vi "ProdaNG.Configurator.vi"() -> ()   [LabVIEW 2016]
uses:
  ProdaNG.Tree.TestViewMode.ctl
  ProdaNG.File.Sequence.ctl
  ProdaNG.Tree.Fglb.Value.ctl
  ProdaNG.File.Step.ctl
  ProdaNG.Configurator.DB.ctl
  ProdaNG.Configurator.Config.ctl
  ProdaNG.Configurator.ResultsTimeSpan.ctl
  Controls/ProdaNG.Product.ctl
  ProdaNG.Configurator.State.ctl
  <vilib>/Utility/error.llb/DialogTypeEnum.ctl
  <vilib>/Utility/miscctls.llb/LVNodeAndColumnTypeDef.ctl
  ProdaNG.Configurator.Glb.vi
panel:
  out "Products":T1[](array[typedef])
  out "DBtime":timestamp
  out "SelectedFile":path
  out "Progress":bool caption="Please wait..."
  out "Hider":bool
  out "PrevTabState":i32
  in  "ButtonResults":bool
  out "SlotInUse":i32
  in  "ButtonTest":bool
  in  "ButtonParts":bool
  out "DB":T2
  out "ProfInfo":string[](array[string])
  in  "TestTreeView":T3
  out "FPref":refnum<vi>
  out "FileContent":T4
  in  "MainTab":enum32{"Parts", "Test", "Results"}(tab)
  in  "ButtonConnect":bool caption="Check"
  out "HiderParts":bool
  in  "ButtonGoToResults":bool
  in  "ButtonGoToTest":bool caption="Accept"
  in  "VariantFilter":string caption="Wabco Part Filter"
  in  "ButtonRefreshTreeProc":bool caption="Refresh"
  in  "ProcTree":string(tree) caption="Found 31 wabco parts"
  out "Identification":T7
  out "Process Found":bool
  in  "color legend 4":u32(colorbox)=16448250 caption="- wabco part"
  in  "color legend 5":u32(colorbox)=12058551 caption="- process"
  in  "color legend 6":u32(colorbox)=16777134 caption="- process step"
  in  "ButtonReloadDB":bool caption="Refresh"
  in  "Configuration":T8={"ShowUnreleased"=TRUE, "Param1"="StepIndex", "ParamStartIdx"=0, "Slots"=1} {"Slots" min=1 max=2; "ParamStartIdx" min=0 max=1}
  in  "TestTree.OpenCloseAll":bool caption="collapse all"
  in  "ButtonSaveToFile":bool
  out "FileInUse":string caption="No file selected"
  in  "ButtonCloseFile":bool
  in  "ButtonExportFile":bool
  in  "ButtonOpenFile":bool
  in  "color legend 1":u32(colorbox)=16448250 caption="- item synchronized"
  in  "color legend 3":u32(colorbox)=16744576 caption="- item value changed"
  in  "color legend 2":u32(colorbox)=16777147 caption="- new item in file (not found in DB)"
  in  "ButtonUnreleaseAll":bool
  in  "ButtonReleaseAll":bool
  in  "ButtonUnrelease":bool
  in  "ButtonRelease":bool
  in  "ButtonDeleteAll":bool
  in  "ButtonAdd":bool
  in  "ButtonEdit":bool
  in  "ButtonDelete":bool
  in  "TestTree":string[](tree)
  in  "ButtonRefreshTestTree":bool
  in  "ResultsAmount":i32=1 caption="Span" min=1 max=100
  in  "ResultsSpan":T9
  in  "Results.TimeTo":timestamp caption="Time To" format="%<%x %X>T"
  in  "Results.TimeFrom":timestamp caption="Time From" format="%<%x %X>T"
  in  "ProductList":i32[](listbox) caption="Products #1"
  in  "color legend 9":u32(colorbox)=16448250 caption="- value ok"
  in  "color legend 8":u32(colorbox)=16744576 caption="- value nok"
  in  "color legend 7":u32(colorbox)=13816530 caption="- value missing"
  in  "ResultsTree":string[](tree)
  in  "ButtonRefreshResultTree":bool
  in  "ProductListSelectAll":enum8{"False", "True", "Mixed"}(c332) caption="All"
  in  "Starthere":bool
  out "Status":string
  out "DBStatus":string
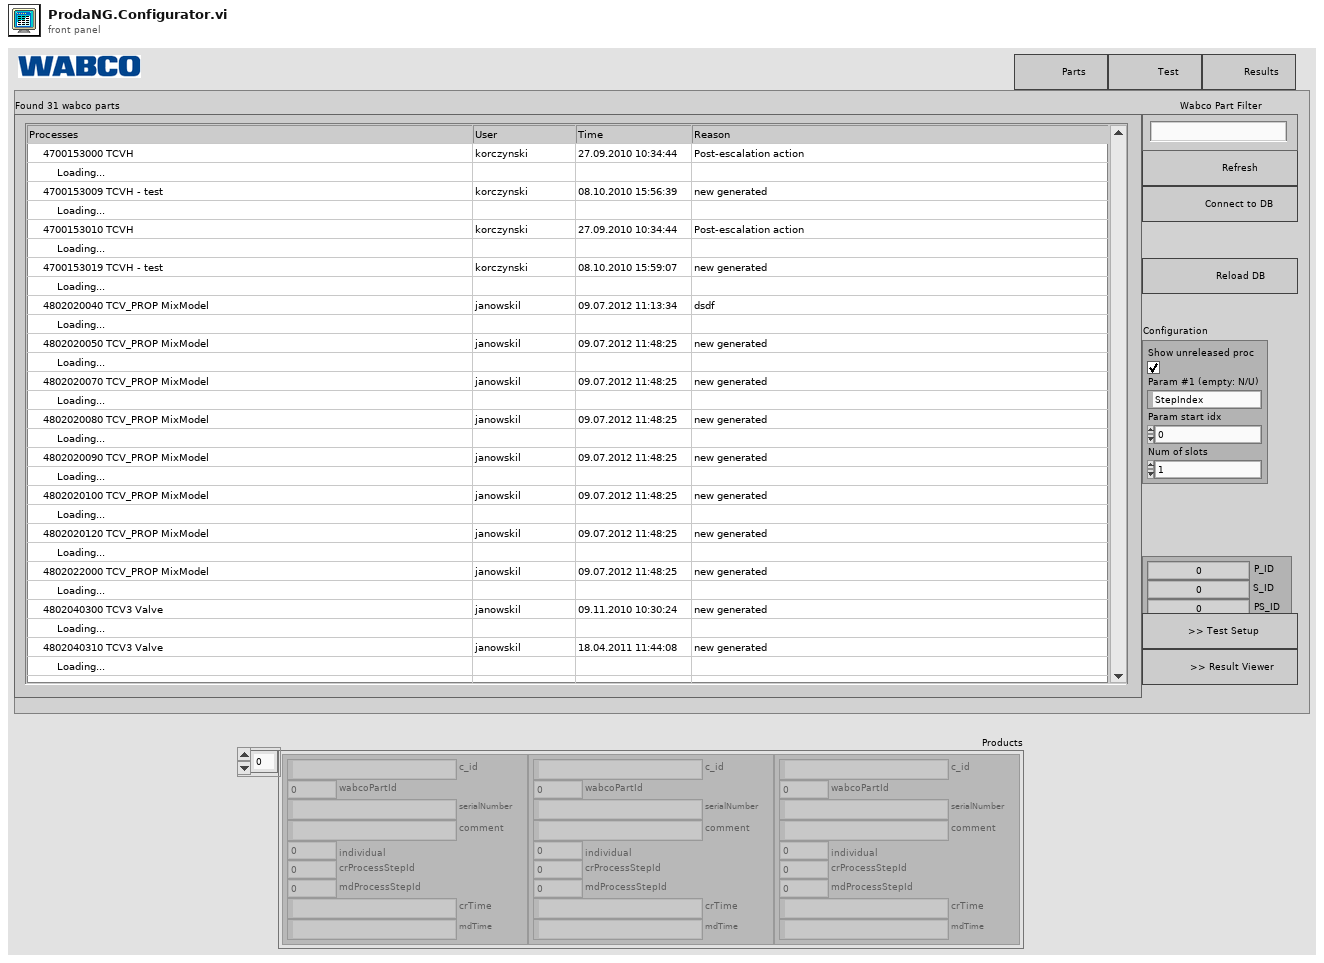
[diagram p1: front panel]
types:
  T1 = typedef "ProdaNG.Product.ctl" = cluster{"c_id":string, "wabcoPartId":i32, "serialNumber":string, "comment":string, "individual":i32, "crProcessStepId":i32, "mdProcessStepId":i32, "crTime":string, "mdTime":string}
  T2 = typedef "ProdaNG.Configurator.DB.ctl" = enum16{"other", "WPL", "WPK"}
  T3 = typedef "ProdaNG.Tree.TestViewMode.ctl" = enum16{"All", "Released", "Unreleased"}
  T4 = typedef "ProdaNG.File.Sequence.ctl" = cluster{"PP":T5[], "TS":T6[]}
  T5 = typedef "ProdaNG.Tree.Fglb.Value.ctl" = cluster{"desc":string, "order":i32, "value1":dbl, "value2":dbl, "unit":i32}
  T6 = typedef "ProdaNG.File.Step.ctl" = cluster{"TS":T5, "TP":T5[], "TV":T5[]}
  T7 = cluster{"P_ID":i32, "S_ID":i32, "PS_ID":i32, "WP_ID":i32}
  T8 = typedef "ProdaNG.Configurator.Config.ctl" = cluster{"ShowUnreleased":bool, "Param1":string, "ParamStartIdx":i32, "Slots":i32}
  T9 = typedef "ProdaNG.Configurator.ResultsTimeSpan.ctl" = enum16{"Custom", "Shift(s)", "Hour(s)", "Day(s)", "Week(s)", "Month(s)"}
  T10 = typedef "ProdaNG.Configurator.State.ctl" = enum16{"Disconnected", "Connected", "ProcessFound"}
  T11 = enum32{"invalid app kind", "Development System", "Run Time System", "Student Edition", "Embedded LabVIEW", "Evaluation", "Custom"}
  T12 = enum8{"Enabled", "Disabled", "Disabled and Grayed Out"}
  T13 = cluster{"processId":i32, "systemId":i32, "processStepId":i32, "wabcoPartId":i32}
  T14 = typedef "DialogTypeEnum.ctl" = enum16{"no dialog", "OK message", "continue or stop message", "auto error handling dialog", "OK message + warnings", "continue/stop + warnings"}
  T15 = typedef "LVNodeAndColumnTypeDef.ctl" = cluster{"Node":string, "Column":i32}
  T16 = enum16{"Custom", "Shift(s)", "Hour(s)", "Day(s)", "Week(s)", "Month(s)"}
  T17 = typedef "LVPositionTypeDef.ctl" = cluster{"Left":i32, "Top":i32}
  T18 = typedef "ProdaNG.ProdutionLine.ctl" = cluster{"i_id":i32, "description":string}
  T19 = typedef "ProdaNG.System.ctl" = cluster{"i_id":i32, "description":string}
  T20 = typedef "ProdaNG.Process.ctl" = cluster{"i_id":i32, "productionLineId":i32, "releaseId":i32, "contentId":string, "previewId":string, "mdReason":string, "mdUser":string, "mdTime":string, "description":string}
  T21 = typedef "ProdaNG.WabcoPart.ctl" = cluster{"i_id":i32, "workCenterId":i32, "contentId":string, "previewId":string, "mdReason":string, "mdUser":string, "mdTime":string, "productName":string, "wabcoNumber":string}
  T22 = typedef "ProdaNG.ProcessStep.ctl" = cluster{"i_id":i32, "processId":i32, "systemId":i32, "releaseId":i32, "processSequence":i32, "limitYellow":dbl, "limitRed":dbl, "mdReason":string, "mdUser":string, "mdTime":string, "filename":string, "transfer":string, "description":string}
  T23 = typedef "ProdaNG.Tree.Fglb.Data.ctl" = cluster{"tag":string, "row":i32, "element":T24, "idx1":i32, "idx2":i32, "file":bool}
  T24 = typedef "ProdaNG.Tree.Fglb.Element.ctl" = enum16{"-", "PP", "TS", "TP", "TV"}
  T25 = typedef "ProdaNG.UnitSimple.ctl" = cluster{"name":string, "i_id":i32}
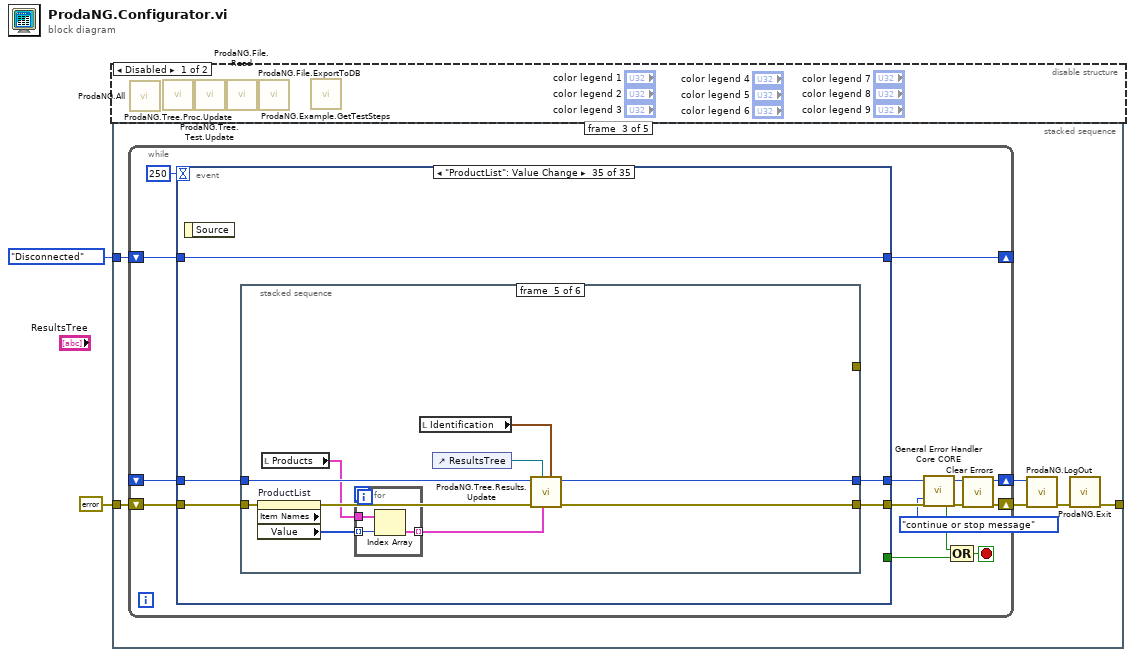
[diagram p0: block diagram]
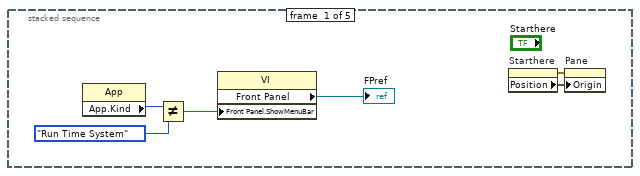
[diagram p2: hidden frame]
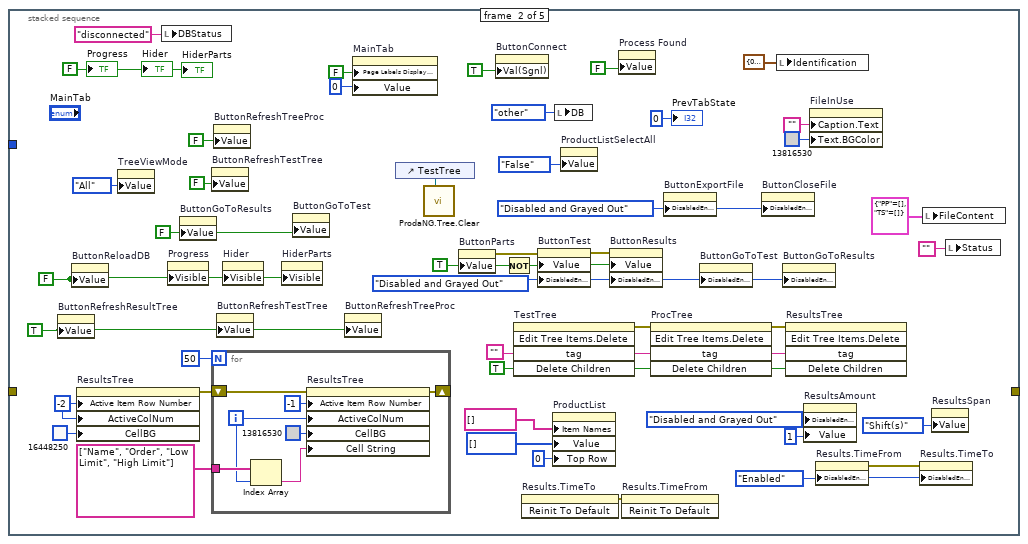
[diagram p3: hidden frame]
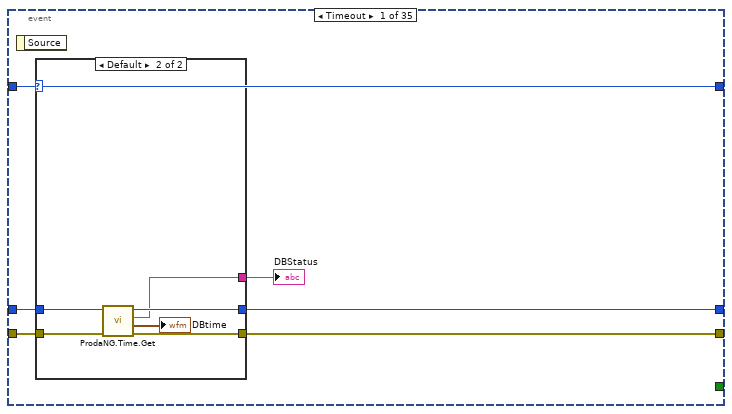
[diagram p4: hidden frame]
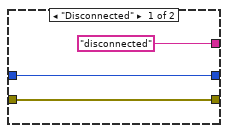
[diagram p5: hidden frame]
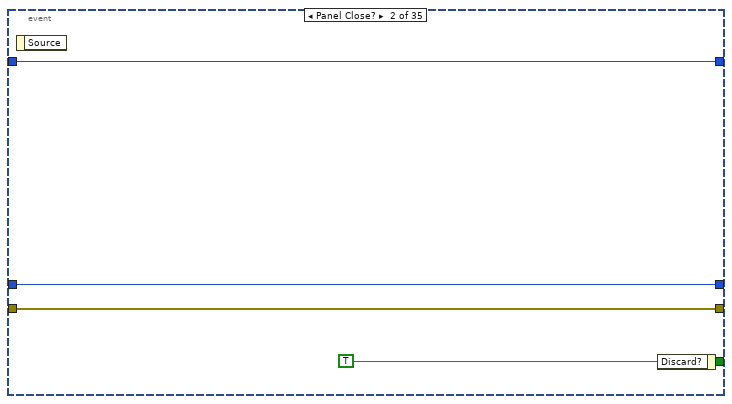
[diagram p6: hidden frame]
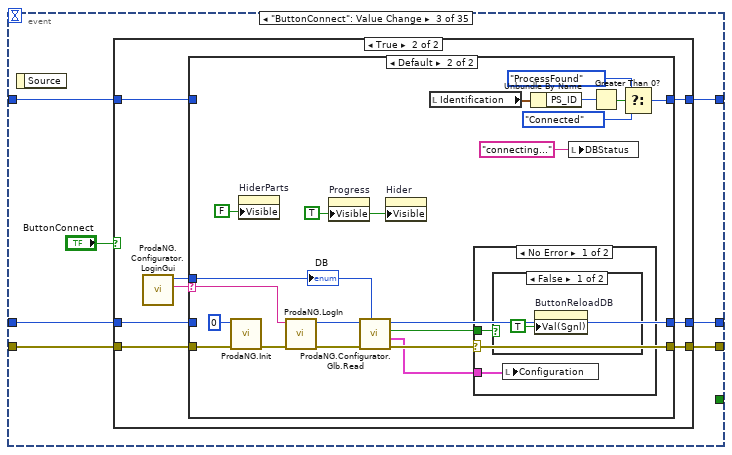
[diagram p7: hidden frame]
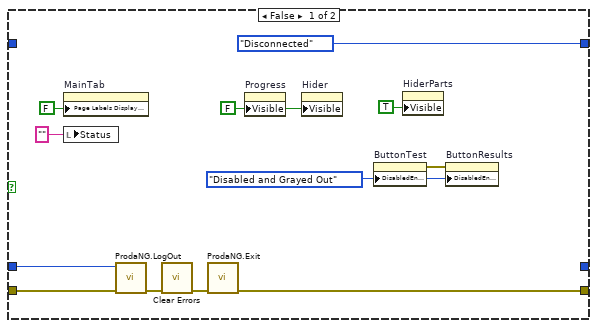
[diagram p8: hidden frame]
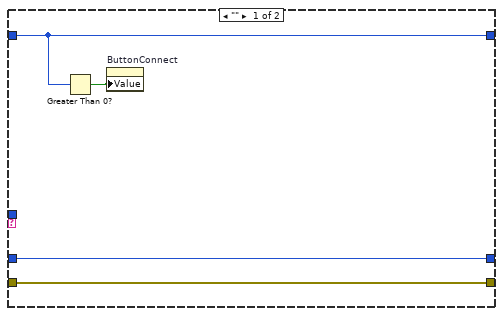
[diagram p9: hidden frame]
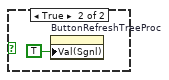
[diagram p10: hidden frame]
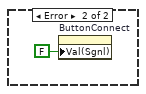
[diagram p11: hidden frame]
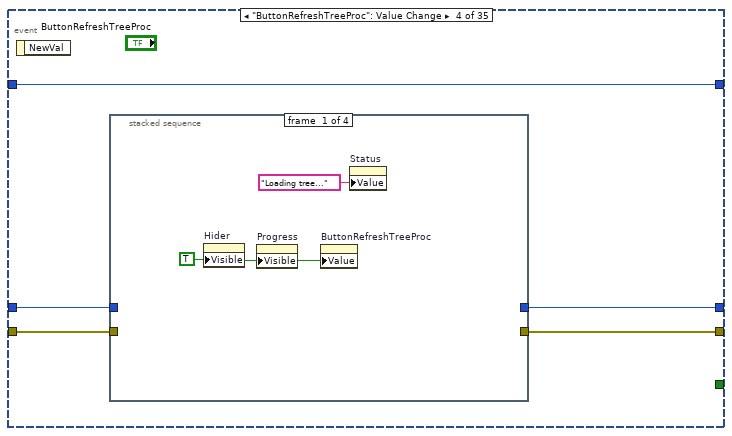
[diagram p12: hidden frame]
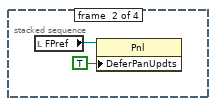
[diagram p13: hidden frame]
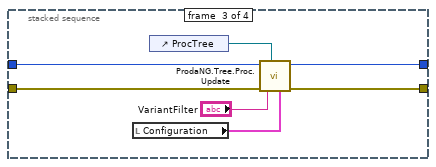
[diagram p14: hidden frame]
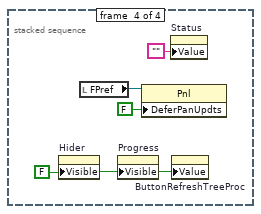
[diagram p15: hidden frame]
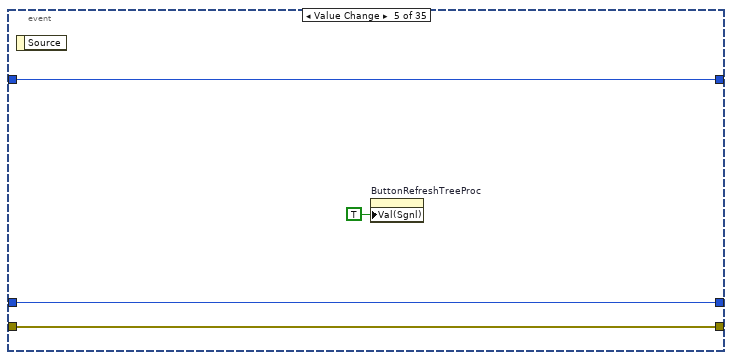
[diagram p16: hidden frame]
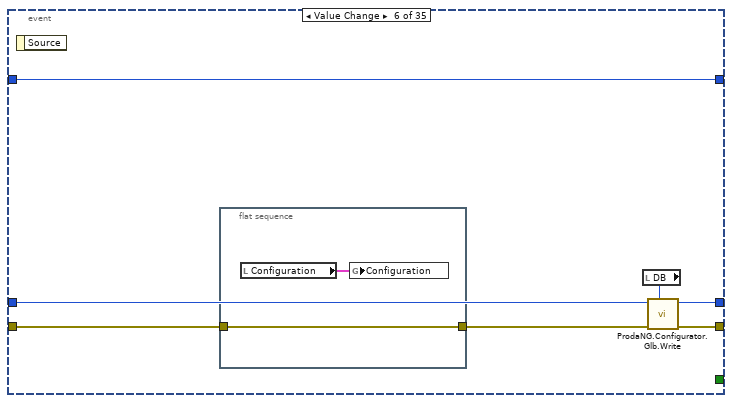
[diagram p17: hidden frame]
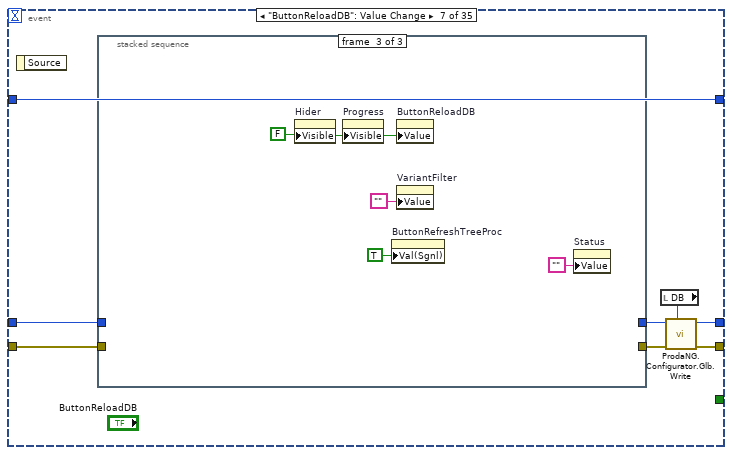
[diagram p18: hidden frame]
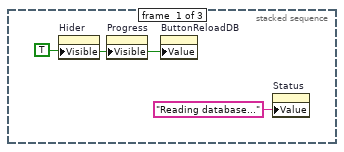
[diagram p19: hidden frame]
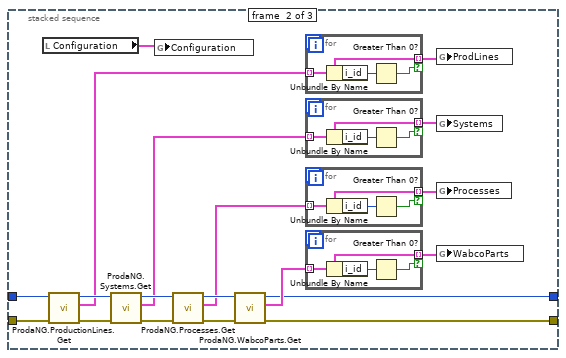
[diagram p20: hidden frame]
diagram:
  n1 = disable-structure shown="Disabled" {
    frame Disabled {
      n2 = call "ProdaNG.All.vi"() -> ()  [unwired: 1 in]
      n3 = call "ProdaNG.Tree.Proc.Update.vi"() -> ()  [unwired: 10 in, 2 out]
      n4 = call "ProdaNG.Tree.Test.Update.vi"() -> ()  [unwired: 8 in, 4 out]
      n5 = call "ProdaNG.File.Read.vi"() -> ()  [unwired: 9 in, 3 out]
      n6 = call "ProdaNG.File.ExportToDB.vi"() -> ()  [unwired: 10 in, 2 out]
      n7 = call "ProdaNG.Example.GetTestSteps.vi"() -> ()  [unwired: 12 in]
    }
    frame Enabled {
    }
  }
  n8 = stacked-sequence {
    tunnel: ProdaNG.Configurator.State."Disconnected" ("State") -> [_ _ w64 _ _]
    tunnel: [_ _ w62 _ _] -> _
    tunnel: errorcluster {"status"=FALSE, "code"=0, "source"=""} ("error out") -> [_ _ w61 _ _]
    frame #0 {
      n9 = property class="App"() -> ("App.Kind"=w8:T11)  [unwired: 2 in, 2 out]
      n10 = Not Equal?(x=w8, y=T11."Run Time System") -> (x != y?=w5:bool)
      n11 = property class="VI"("Front Panel.ShowMenuBar"=w5) -> ("Front Panel"=→"FPref":refnum<vi>)  [unwired: 2 in, 2 out]
      n12 = property on="Starthere" class="Bool (strict)"() -> (error out=w4:errorcluster, "Position"=w3:T17)  [unwired: 2 in, 1 out]
      n13 = property on="Pane" class="Pane"(error in=w4, "Origin"=w3) -> ()  [unwired: 1 in, 2 out]
    }
    frame #1 {
      w11 = T12."Enabled" ("Disabled")
      w15 = TRUE ("Value (Signaling)")
      w21 = -2 ("Active Item:Row Number")
      w26 = TRUE ("Delete Children?")
      w27 = ""
      w31 = FALSE ("Progress")
      w32 = FALSE ("ButtonGoToResults")
      w34 = T12."Disabled and Grayed Out" ("Disabled")
      w39 = TRUE ("ButtonPartList")
      w30 = FALSE ("Visible")
      w47 = T12."Disabled and Grayed Out" ("Disabled")
      n14 = property on="ButtonRefreshResultTree" class="Bool (strict)"("Value"=w15) -> ()  [unwired: 2 in, 2 out]
      n15 = property on="ButtonReloadDB" class="Bool (strict)"("Value"=w30) -> ()  [unwired: 2 in, 2 out]
      n16 = property on="ResultsTree" class="Tree (strict)"("Active Item Row Number"=w21, "ActiveColNum"=w21, "CellBG"=u32 16448250) -> (error out=w22:errorcluster)  [unwired: 2 in, 1 out]
      n17 = property on="TreeViewMode" class="Enum (strict)"("Value"=ProdaNG.Tree.TestViewMode."All" ("TreeViewMode")) -> ()  [unwired: 2 in, 2 out]
      n18 = local write "DBStatus"("disconnected" ("string")) -> ()
      n19 = property on="Progress" class="Bool (strict)"("Visible"=w30) -> ()  [unwired: 2 in, 2 out]
      n20 = property on="ButtonGoToResults" class="Bool (strict)"("Value"=w32) -> ()  [unwired: 2 in, 2 out]
      n21 = property on="ButtonRefreshTestTree" class="Bool (strict)"("Value"=FALSE ("ButtonRefreshSystem")) -> ()  [unwired: 2 in, 2 out]
      n22 = for {
        N: 50 -> [_]
        tunnel: string[] ["Name", "Order", "Low Limit", "High Limit"] -> [w57]
        shift-right: [w55] -> _
        shift-left: w22 -> [w60]
        i -> [w54]
        n23 = Index Array(array=w57, index=w54) -> (element=w56:string)
        n24 = property on="ResultsTree" class="Tree (strict)"(error in=w60, "Active Item Row Number"=-1 ("Active Item:Row Number"), "ActiveColNum"=w54, "CellBG"=u32 13816530, "Cell String"=w56) -> (error out=w55:errorcluster)  [unwired: 1 in, 1 out]
      }
      n25 = property on="ButtonRefreshTreeProc" class="Bool (strict)"("Value"=FALSE ("Value (Signaling)")) -> ()  [unwired: 2 in, 2 out]
      n26 = property on="ButtonRefreshTestTree" class="Bool (strict)"("Value"=w15) -> ()  [unwired: 2 in, 2 out]
      n27 = property on="Hider" class="Bool (strict)"("Visible"=w30) -> ()  [unwired: 2 in, 2 out]
      n28 = property on="HiderParts" class="Bool (strict)"("Visible"=w30) -> ()  [unwired: 2 in, 2 out]
      n29 = property on="ButtonGoToTest" class="Bool (strict)"("Value"=w32) -> ()  [unwired: 2 in, 2 out]
      n30 = property on="ButtonRefreshTreeProc" class="Bool (strict)"("Value"=w15) -> ()  [unwired: 2 in, 2 out]
      n31 = property on="MainTab" class="TabCtl (strict)"("Page Labels Display Visible?"=FALSE, "Value"=0) -> ()  [unwired: 2 in, 2 out]
      n32 = control-ref of="TestTree"() -> (w51:refnum<vi>)
      n33 = call "ProdaNG.Tree.Clear.vi"("TestStepsTree"=w51) -> ()  [unwired: 10 in, 1 out]
      n34 = property on="ButtonParts" class="Bool (strict)"("Value"=w39) -> (error out=w38:errorcluster)  [unwired: 2 in, 1 out]
      n35 = property on="ButtonConnect" class="Bool (strict)"("Val(Sgnl)"=TRUE ("ButtonConnect")) -> ()  [unwired: 2 in, 2 out]
      n36 = Not(x=w39) -> (.not. x?=w36:bool)
      n37 = invoke on="TestTree" class="Tree (strict)" method="Edit Tree Items.Delete"("tag"=w27, "Delete Children"=w26) -> (error out=w29:errorcluster)  [unwired: 3 in, 4 out]
      n38 = invoke on="Results.TimeTo" class="AbsTime (strict)" method="Reinit To Default"() -> (error out=w9:errorcluster)  [unwired: 3 in, 2 out]
      n39 = property on="ButtonTest" class="Bool (strict)"(error in=w38, "Value"=w36, "DisabledEnum"=w34) -> (error out=w37:errorcluster)  [unwired: 1 in, 1 out]
      n40 = property on="ProductList" class="LstBox (strict)"("Item Names"=string[] [], "Value"=i32[] [] ("ProductList"), "Top Row"=0) -> ()  [unwired: 2 in, 2 out]
      n41 = local write "DB"(ProdaNG.Configurator.DB."other" ("DB")) -> ()
      n42 = property on="ProductListSelectAll" class="MixedCheckbox (strict)"("Value"=enum8{"False", "True", "Mixed"}."False" ("Mixed Checkbox")) -> ()  [unwired: 2 in, 2 out]
      n43 = property on="ButtonResults" class="Bool (strict)"(error in=w37, "Value"=w36, "DisabledEnum"=w34) -> ()  [unwired: 1 in, 2 out]
      n44 = property on="Process Found" class="Bool (strict)"("Value"=FALSE ("Visible")) -> ()  [unwired: 2 in, 2 out]
      n45 = invoke on="Results.TimeFrom" class="AbsTime (strict)" method="Reinit To Default"(error in=w9) -> ()  [unwired: 2 in, 3 out]
      n46 = invoke on="ProcTree" class="Tree (strict)" method="Edit Tree Items.Delete"(error in=w29, "tag"=w27, "Delete Children"=w26) -> (error out=w28:errorcluster)  [unwired: 2 in, 4 out]
      n47 = property on="ButtonExportFile" class="Bool (strict)"("DisabledEnum"=w47) -> ()  [unwired: 2 in, 2 out]
      n48 = property on="ButtonGoToTest" class="Bool (strict)"("DisabledEnum"=w34) -> ()  [unwired: 2 in, 2 out]
      n49 = property on="ButtonCloseFile" class="Bool"("DisabledEnum"=w47) -> ()  [unwired: 2 in, 2 out]
      n50 = local write "Identification"(T13 {"processId"=0, "systemId"=0, "processStepId"=0, "wabcoPartId"=0} ("Identification")) -> ()
      n51 = property on="ButtonGoToResults" class="Bool (strict)"("DisabledEnum"=w34) -> ()  [unwired: 2 in, 2 out]
      n52 = invoke on="ResultsTree" class="Tree (strict)" method="Edit Tree Items.Delete"(error in=w28, "tag"=w27, "Delete Children"=w26) -> ()  [unwired: 2 in, 5 out]
      n53 = property on="ResultsAmount" class="DigNum (strict)"("DisabledEnum"=T12."Disabled and Grayed Out" ("Disabled"), "Value"=1 ("ResultsAmount")) -> ()  [unwired: 2 in, 2 out]
      n54 = property on="FileInUse" class="Str"("Caption.Text"="", "Text.BGColor"=u32 13816530) -> ()  [unwired: 2 in, 2 out]
      n55 = property on="Results.TimeFrom" class="AbsTime (strict)"("DisabledEnum"=w11) -> (error out=w12:errorcluster)  [unwired: 2 in, 1 out]
      n56 = property on="Results.TimeTo" class="AbsTime (strict)"(error in=w12, "DisabledEnum"=w11) -> ()  [unwired: 1 in, 2 out]
      n57 = local write "FileContent"(T4 {"PP"=[], "TS"=[]} ("Seq")) -> ()
      n58 = property on="ResultsSpan" class="Enum (strict)"("Value"=ProdaNG.Configurator.ResultsTimeSpan."Shift(s)" ("ResultsSpan")) -> ()  [unwired: 2 in, 2 out]
      n59 = local write "Status"("") -> ()
      "PrevTabState" <- 0 ("PrevTabState")
      "Hider" <- w31
      "Progress" <- w31
      "HiderParts" <- w31
    }
    frame #2 {
      n60 = while {
        shift-right: [w74] -> w65
        shift-left: w61 -> [w78]
        shift-right: [w79] -> w66
        shift-left: _ -> [w77]
        shift-right: [w67] -> _
        shift-left: w64 -> [w75]
        stop <- w70 stop-if-true
        n61 = event shown="[34] \"ProductList\": Value Change" {
          selector: _ -> [_ _ _ _ _ _ _ _ _ _ _ _ _ _ _ _ _ _ _ _ _ _ _ _ _ _ _ _ _ _ _ _ _ _ _]
          dyn-events: _ -> [_ _ _ _ _ _ _ _ _ _ _ _ _ _ _ _ _ _ _ _ _ _ _ _ _ _ _ _ _ _ _ _ _ _ _]
          timeout: 250 -> [_ _ _ _ _ _ _ _ _ _ _ _ _ _ _ _ _ _ _ _ _ _ _ _ _ _ _ _ _ _ _ _ _ _ _]
          tunnel: [w83 w95 w104 w156 w175 w180 w189 w234 w243 w251 w266 w275 w293 w350 w362 w372 w432 w456 w466 w510 w554 w598 w648 w684 w727 w764 w803 w852 w860 w890 w935 w1022 w1031 w1033 w1046] -> w79
          tunnel: w78 -> [w85 w96 w105 w155 w176 w179 w191 w235 w244 w252 w267 w276 w296 w351 w363 w366 w446 w457 w465 w509 w553 w597 w642 w681 w730 w767 w806 w853 w861 w891 w929 w1021 w1030 w1034 w1048]
          tunnel: w77 -> [w84 w95 w101 w157 w175 w180 w190 w234 w243 w251 w266 w275 w295 w350 w362 w370 w432 w456 w468 w512 w556 w600 w641 w678 w729 w766 w803 w852 w862 w892 w933 w1022 w1031 w1033 w1047]
          tunnel: [w80 w96 w103 w154 w176 w181 w187 w235 w244 w252 w267 w276 w294 w351 w363 w365 w430 w457 w467 w511 w555 w599 w649 w685 w728 w765 w805 w853 w859 w903 w928 w1021 w1030 w1034 w1045] -> w73
          tunnel: [w82 w98 w100 w158 w177 w183 w192 w237 w245 w253 w268 w284 w297 ProdaNG.Configurator.State."ProcessFound" ("State") ProdaNG.Configurator.State."ProcessFound" ("State") w371 w447 w458 w459 w503 w547 w591 w647 w683 w726 w763 w809 w856 w863 w904 w934 w1023 w1032 w1038 w1049] -> w67
          tunnel: w75 -> [w82 w98 w99 w158 w177 w183 w192 w237 w245 w253 w268 w284 w297 _ _ w371 w447 w458 w459 w503 w547 w591 w647 w683 w726 w763 w809 w856 w863 w904 w934 w1023 w1032 w1038 w1049]
          tunnel: [_ w97 _ _ _ _ _ _ _ _ _ _ _ _ _ _ _ _ _ _ _ _ _ _ _ _ _ _ _ _ _ _ _ _ _] -> w71
          event Timeout {
            n62 = event-data() -> ()  [unwired: 1 in, 1 out]
            n63 = case shown="Default" w82 {
              tunnel: w85 -> [w88 w94]
              tunnel: [w88 w93] -> w80
              tunnel: w84 -> [w87 w92]
              tunnel: [w87 w91] -> w83
              tunnel: ["disconnected" ("string") w90] -> w81
              frame "Disconnected" {
              }
              frame Default {
                n64 = call "ProdaNG.Time.Get.vi"("error in"=w94, "dbHandleIn"=w92) -> ("error out"=w93:errorcluster, "time"=→"DBtime":timestamp, "timeStr"=w90:string, "dbHandle"=w91:i32)  [unwired: 5 in]
              }
            }
            "DBStatus" <- w81
          }
          event Panel Close? {
            w97 = TRUE ("Discard?")
            n65 = event-data() -> ()  [unwired: 1 in, 1 out]
            n66 = event-data("Discard?"=w97) -> ()  [unwired: 1 in, 1 out]
          }
          event "ButtonConnect": Value Change {
            n67 = event-data() -> ()  [unwired: 1 in, 1 out]
            n68 = case shown="True" "ButtonConnect" {
              tunnel: w105 -> [w116 w125]
              tunnel: [_ w123] -> w104
              tunnel: [w115 w124] -> w103
              tunnel: w101 -> [w114 w121]
              tunnel: [ProdaNG.Configurator.State."Disconnected" ("State") w119] -> w100
              tunnel: w99 -> [_ w120]
              frame False {
                w106 = FALSE ("Visible")
                w108 = T12."Disabled and Grayed Out" ("Disabled")
                n69 = property on="MainTab" class="TabCtl (strict)"("Page Labels Display Visible?"=FALSE) -> ()  [unwired: 2 in, 2 out]
                n70 = local write "Status"("" ("Status")) -> ()
                n71 = call "ProdaNG.LogOut.vi"("error in"=w116, "dbHandleIn"=w114) -> ("error out"=w117:errorcluster)  [unwired: 9 in]
                n72 = call <vilib>:"Clear Errors.vi"("error in (no error)"=w117) -> ("error out"=w109:errorcluster)  [unwired: 5 in, 1 out]
                n73 = call "ProdaNG.Exit.vi"("error in (no error)"=w109) -> ("error out"=w115:errorcluster)  [unwired: 10 in]
                n74 = property on="Progress" class="Bool (strict)"("Visible"=w106) -> ()  [unwired: 2 in, 2 out]
                n75 = property on="Hider" class="Bool (strict)"("Visible"=w106) -> ()  [unwired: 2 in, 2 out]
                n76 = property on="ButtonTest" class="Bool (strict)"("DisabledEnum"=w108) -> (error out=w107:errorcluster)  [unwired: 2 in, 1 out]
                n77 = property on="HiderParts" class="Bool (strict)"("Visible"=TRUE) -> ()  [unwired: 2 in, 2 out]
                n78 = property on="ButtonResults" class="Bool (strict)"(error in=w107, "DisabledEnum"=w108) -> ()  [unwired: 1 in, 2 out]
              }
              frame True {
                n79 = call "ProdaNG.Configurator.LoginGui.vi"() -> ("ConnectionString"=w122:string, "DB"=w118:T2)  [unwired: 10 in]
                n80 = case shown="Default" w122 {
                  selector: w122 -> [_ w145]
                  tunnel: w125 -> [w128 w146]
                  tunnel: [w128 w137] -> w124
                  tunnel: [w129 w131] -> w123
                  tunnel: w121 -> [w129 _]
                  tunnel: w120 -> [w127 _]
                  tunnel: [w127 w139] -> w119
                  tunnel: w118 -> [_ w138]
                  frame "" {
                    n81 = Greater Than 0?(x=w127) -> (x > 0?=w126:bool)
                    n82 = property on="ButtonConnect" class="Bool (strict)"("Value"=w126) -> ()  [unwired: 2 in, 2 out]
                  }
                  frame Default {
                    w134 = TRUE ("Visible")
                    n83 = call "ProdaNG.Init.vi"("error in (no error)"=w146, "numContexts (0: unlimited)"=0 ("numContexts")) -> ("error out"=w147:errorcluster)  [unwired: 9 in]
                    n84 = property on="HiderParts" class="Bool (strict)"("Visible"=FALSE) -> ()  [unwired: 2 in, 2 out]
                    n85 = call "ProdaNG.LogIn.vi"("error in"=w147, "ConnectionString"=w145) -> ("error out"=w132:errorcluster, "dbHandle"=w131:i32)  [unwired: 7 in, 1 out]
                    n86 = property on="Progress" class="Bool (strict)"("Visible"=w134) -> ()  [unwired: 2 in, 2 out]
                    n87 = call "ProdaNG.Configurator.Glb.Read.vi"("DB"=w138, "error in (no error)"=w132) -> ("error out"=w137:errorcluster, "Configuration"=w130:T8, "Data found"=w136:bool)  [unwired: 7 in]
                    n88 = property on="Hider" class="Bool (strict)"("Visible"=w134) -> ()  [unwired: 2 in, 2 out]
                    n89 = local read "Identification"() -> (w140:T7)
                    n90 = case shown="No Error" w137 {
                      tunnel: w136 -> [w150 _]
                      tunnel: w130 -> [w149 _]
                      frame No Error {
                        n91 = case shown="False" w150 {
                          frame False {
                            n92 = property on="ButtonReloadDB" class="Bool (strict)"("Val(Sgnl)"=TRUE ("Value (Signaling)")) -> ()  [unwired: 2 in, 2 out]
                          }
                          frame True {
                            n93 = property on="ButtonRefreshTreeProc" class="Bool (strict)"("Val(Sgnl)"=TRUE ("Value (Signaling)")) -> ()  [unwired: 2 in, 2 out]
                          }
                        }
                        n94 = local write "Configuration"(w149) -> ()
                      }
                      frame Error {
                        n95 = property on="ButtonConnect" class="Bool (strict)"("Val(Sgnl)"=FALSE ("Value (Signaling)")) -> ()  [unwired: 2 in, 2 out]
                      }
                    }
                    n96 = Unbundle By Name(w140) -> ("PS_ID"=w141:i32)
                    n97 = local write "DBStatus"("connecting..." ("Front Panel Window:Title")) -> ()
                    n98 = Greater Than 0?(x=w141) -> (x > 0?=w142:bool)
                    n99 = Select(t=ProdaNG.Configurator.State."ProcessFound" ("State"), s=w142, f=ProdaNG.Configurator.State."Connected" ("State")) -> (s? t:f=w139:T10)
                    "DB" <- w138
                  }
                }
              }
            }
          }
          event "ButtonRefreshTreeProc": Value Change {
            n100 = event-data() -> ()  [unwired: 1 in, 1 out]
            n101 = stacked-sequence {
              tunnel: w157 -> [_ _ w169 _]
              tunnel: [_ _ w168 _] -> w156
              tunnel: w155 -> [_ _ w165 _]
              tunnel: [_ _ w164 _] -> w154
              frame #0 {
                w159 = TRUE ("Visible")
                n102 = property on="Hider" class="Bool (strict)"("Visible"=w159) -> ()  [unwired: 2 in, 2 out]
                n103 = property on="Progress" class="Bool (strict)"("Visible"=w159) -> ()  [unwired: 2 in, 2 out]
                n104 = property on="ButtonRefreshTreeProc" class="Bool (strict)"("Value"=w159) -> ()  [unwired: 2 in, 2 out]
                n105 = property on="Status" class="Str"("Value"="Loading tree..." ("Status")) -> ()  [unwired: 2 in, 2 out]
              }
              frame #1 {
                n106 = local read "FPref"() -> (w161:refnum<vi>)
                n107 = property class="Pnl"(reference=w161, "DeferPanUpdts"=TRUE ("Defer Panel Updates")) -> ()  [unwired: 1 in, 2 out]
              }
              frame #2 {
                n108 = local read "Configuration"() -> (w163:T8)
                n109 = control-ref of="ProcTree"() -> (w167:refnum<vi>)
                n110 = call "ProdaNG.Tree.Proc.Update.vi"("Configuration"=w163, "VariantFilter"="VariantFilter", "Tree"=w167, "error in (no error)"=w165, "dbHandle in"=w169) -> ("error out"=w164:errorcluster, "dbHandle out"=w168:i32)  [unwired: 5 in]
              }
              frame #3 {
                w170 = FALSE ("Visible")
                n111 = property on="Hider" class="Bool (strict)"("Visible"=w170) -> ()  [unwired: 2 in, 2 out]
                n112 = local read "FPref"() -> (w172:refnum<vi>)
                n113 = property on="Progress" class="Bool (strict)"("Visible"=w170) -> ()  [unwired: 2 in, 2 out]
                n114 = property class="Pnl"(reference=w172, "DeferPanUpdts"=FALSE ("Defer Panel Updates")) -> ()  [unwired: 1 in, 2 out]
                n115 = property on="Status" class="Str"("Value"="") -> ()  [unwired: 2 in, 2 out]
                n116 = property on="ButtonRefreshTreeProc" class="Bool (strict)"("Value"=w170) -> ()  [unwired: 2 in, 2 out]
              }
            }
          }
          event Value Change {
            n117 = event-data() -> ()  [unwired: 1 in, 1 out]
            n118 = property on="ButtonRefreshTreeProc" class="Bool (strict)"("Val(Sgnl)"=TRUE ("Value (Signaling)")) -> ()  [unwired: 2 in, 2 out]
          }
          event Value Change {
            n119 = event-data() -> ()  [unwired: 1 in, 1 out]
            n120 = flat-sequence {
              tunnel: w179 -> [w184]
              tunnel: [w184] -> w178
              frame #0 {
                n121 = local read "Configuration"() -> (w185:T8)
                n122 = global write "ProdaNG.Configurator.Glb.vi" "Configuration"(w185) -> ()
              }
            }
            n123 = local read "DB"() -> (w182:T2)
            n124 = call "ProdaNG.Configurator.Glb.Write.vi"("DB"=w182, "error in (no error)"=w178) -> ("error out"=w181:errorcluster)  [unwired: 9 in]
          }
          event "ButtonReloadDB": Value Change {
            n125 = event-data() -> ()  [unwired: 1 in, 1 out]
            n126 = stacked-sequence {
              tunnel: w191 -> [_ w204 _]
              tunnel: w190 -> [_ w210 _]
              tunnel: [_ w209 _] -> w189
              tunnel: [_ w208 _] -> w188
              frame #0 {
                w193 = TRUE ("Visible")
                n127 = property on="Hider" class="Bool (strict)"("Visible"=w193) -> ()  [unwired: 2 in, 2 out]
                n128 = property on="Progress" class="Bool (strict)"("Visible"=w193) -> ()  [unwired: 2 in, 2 out]
                n129 = property on="ButtonReloadDB" class="Bool (strict)"("Value"=w193) -> ()  [unwired: 2 in, 2 out]
                n130 = property on="Status" class="Str"("Value"="Reading database..." ("Status")) -> ()  [unwired: 2 in, 2 out]
              }
              frame #1 {
                n131 = local read "Configuration"() -> (w195:T8)
                n132 = call "ProdaNG.ProductionLines.Get.vi"("error in (no error)"=w204, "dbHandleIn"=w210) -> ("error out"=w203:errorcluster, "ProdLines"=w202:T18[], "dbHandle"=w205:i32)  [unwired: 7 in]
                n133 = call "ProdaNG.Systems.Get.vi"("error in (no error)"=w203, "dbHandleIn"=w205) -> ("error out"=w199:errorcluster, "Systems"=w211:T19[], "dbHandle"=w212:i32)  [unwired: 7 in]
                n134 = global write "ProdaNG.Configurator.Glb.vi" "Configuration"(w195) -> ()
                n135 = call "ProdaNG.Processes.Get.vi"("error in (no error)"=w199, "dbHandleIn"=w212) -> ("error out"=w198:errorcluster, "Processes"=w196:T20[], "dbHandle"=w200:i32)  [unwired: 7 in]
                n136 = call "ProdaNG.WabcoParts.Get.vi"("error in (no error)"=w198, "dbHandleIn"=w200) -> ("error out"=w208:errorcluster, "WabcoParts"=w213:T21[], "dbHandle"=w209:i32)  [unwired: 7 in]
                n137 = for {
                  tunnel: w202 -> [w219] mode=indexing
                  tunnel: [w219] -> w201 mode=indexing if=w217
                  n138 = Unbundle By Name(w219) -> ("i_id"=w218:i32)
                  n139 = Greater Than 0?(x=w218) -> (x > 0?=w217:bool)
                }
                n140 = for {
                  tunnel: w211 -> [w225] mode=indexing
                  tunnel: [w225] -> w206 mode=indexing if=w223
                  n141 = Unbundle By Name(w225) -> ("i_id"=w224:i32)
                  n142 = Greater Than 0?(x=w224) -> (x > 0?=w223:bool)
                }
                n143 = for {
                  tunnel: w196 -> [w216] mode=indexing
                  tunnel: [w216] -> w197 mode=indexing if=w214
                  n144 = Unbundle By Name(w216) -> ("i_id"=w215:i32)
                  n145 = Greater Than 0?(x=w215) -> (x > 0?=w214:bool)
                }
                n146 = for {
                  tunnel: w213 -> [w222] mode=indexing
                  tunnel: [w222] -> w207 mode=indexing if=w220
                  n147 = Unbundle By Name(w222) -> ("i_id"=w221:i32)
                  n148 = Greater Than 0?(x=w221) -> (x > 0?=w220:bool)
                }
                n149 = global write "ProdaNG.Configurator.Glb.vi" "ProdLines"(w201) -> ()
                n150 = global write "ProdaNG.Configurator.Glb.vi" "Systems"(w206) -> ()
                n151 = global write "ProdaNG.Configurator.Glb.vi" "Processes"(w197) -> ()
                n152 = global write "ProdaNG.Configurator.Glb.vi" "WabcoParts"(w207) -> ()
              }
              frame #2 {
                w226 = FALSE ("Visible")
                n153 = property on="Hider" class="Bool (strict)"("Visible"=w226) -> ()  [unwired: 2 in, 2 out]
                n154 = property on="Progress" class="Bool (strict)"("Visible"=w226) -> ()  [unwired: 2 in, 2 out]
                n155 = property on="ButtonRefreshTreeProc" class="Bool (strict)"("Val(Sgnl)"=TRUE ("Value (Signaling)")) -> ()  [unwired: 2 in, 2 out]
                n156 = property on="ButtonReloadDB" class="Bool (strict)"("Value"=w226) -> ()  [unwired: 2 in, 2 out]
                n157 = property on="VariantFilter" class="Str"("Value"="") -> ()  [unwired: 2 in, 2 out]
                n158 = property on="Status" class="Str"("Value"="") -> ()  [unwired: 2 in, 2 out]
              }
            }
            n159 = local read "DB"() -> (w186:T2)
            n160 = call "ProdaNG.Configurator.Glb.Write.vi"("DB"=w186, "error in (no error)"=w188) -> ("error out"=w187:errorcluster)  [unwired: 9 in]
          }
          event "ButtonParts": Value Change {
            w233 = TRUE ("ButtonPartList")
            n161 = event-data() -> ()  [unwired: 1 in, 1 out]
            n162 = property on="ButtonParts" class="Bool (strict)"("Value"=w233) -> (error out=w232:errorcluster)  [unwired: 2 in, 1 out]
            n163 = Not(x=w233) -> (.not. x?=w230:bool)
            n164 = property on="MainTab" class="TabCtl (strict)"("Value"=0) -> ()  [unwired: 2 in, 2 out]
            n165 = property on="ButtonTest" class="Bool (strict)"(error in=w232, "Value"=w230) -> (error out=w231:errorcluster)  [unwired: 1 in, 1 out]
            n166 = property on="ButtonResults" class="Bool (strict)"(error in=w231, "Value"=w230) -> ()  [unwired: 1 in, 2 out]
          }
          event "ButtonTest": Value Change {
            w242 = TRUE ("ButtonPartList")
            w238 = 1
            n167 = event-data() -> ()  [unwired: 1 in, 1 out]
            n168 = property on="ButtonTest" class="Bool (strict)"("Value"=w242) -> (error out=w241:errorcluster)  [unwired: 2 in, 1 out]
            n169 = Not(x=w242) -> (.not. x?=w239:bool)
            n170 = property on="ButtonParts" class="Bool (strict)"(error in=w241, "Value"=w239) -> (error out=w240:errorcluster)  [unwired: 1 in, 1 out]
            n171 = property on="MainTab" class="TabCtl (strict)"("Value"=w238) -> ()  [unwired: 2 in, 2 out]
            n172 = property on="ButtonResults" class="Bool (strict)"(error in=w240, "Value"=w239) -> ()  [unwired: 1 in, 2 out]
            n173 = local write "PrevTabState"(w238) -> ()
          }
          event "ButtonResults": Value Change {
            w250 = TRUE ("ButtonPartList")
            w246 = 2
            n174 = event-data() -> ()  [unwired: 1 in, 1 out]
            n175 = property on="ButtonResults" class="Bool (strict)"("Value"=w250) -> (error out=w249:errorcluster)  [unwired: 2 in, 1 out]
            n176 = Not(x=w250) -> (.not. x?=w247:bool)
            n177 = property on="ButtonParts" class="Bool (strict)"(error in=w249, "Value"=w247) -> (error out=w248:errorcluster)  [unwired: 1 in, 1 out]
            n178 = property on="MainTab" class="TabCtl (strict)"("Value"=w246) -> ()  [unwired: 2 in, 2 out]
            n179 = property on="ButtonTest" class="Bool (strict)"(error in=w248, "Value"=w247) -> ()  [unwired: 1 in, 2 out]
            n180 = local write "PrevTabState"(w246) -> ()
          }
          event "ProcTree": Value Change {
            n181 = event-data() -> ("CtlRef"=w263:refnum<vi>, "NewVal"=w259:string)  [unwired: 1 in]
            n182 = call "ProdaNG.Tree.Proc.GetTag.vi"("Tree"=w263, "Tag"=w259) -> ("Process Found"=w260:bool, "Identification"=→"Identification":T7, "ProfInfo"=→"ProfInfo":string[], "SlotNo"=→"SlotInUse":i32)  [unwired: 5 in, 1 out]
            "Process Found" <- w260
            n183 = Select(t=T12."Enabled" ("Disabled"), s=w260, f=T12."Disabled and Grayed Out" ("Disabled")) -> (s? t:f=w255:T12)
            n184 = property on="ButtonTest" class="Bool (strict)"("DisabledEnum"=w255) -> (error out=w257:errorcluster)  [unwired: 2 in, 1 out]
            n185 = property on="ButtonResults" class="Bool (strict)"(error in=w257, "DisabledEnum"=w255) -> (error out=w254:errorcluster)  [unwired: 1 in, 1 out]
            n186 = property on="ButtonGoToTest" class="Bool (strict)"(error in=w254, "DisabledEnum"=w255) -> (error out=w256:errorcluster)  [unwired: 1 in, 1 out]
            n187 = property on="ButtonGoToResults" class="Bool (strict)"(error in=w256, "DisabledEnum"=w255) -> ()  [unwired: 1 in, 2 out]
          }
          event "ProcTree": Double Click {
            n188 = event-data() -> ("CtlRef"=w283:refnum<vi>, "Tag"=w278:string)  [unwired: 1 in]
            n189 = call "ProdaNG.Tree.Proc.GetTag.vi"("Tree"=w283, "Tag"=w278) -> ("Process Found"=w277:bool, "Identification"=w282:T7, "ProfInfo"=w281:string[], "SlotNo"=w274:i32)  [unwired: 5 in, 1 out]
            n190 = local write "SlotInUse"(w274) -> ()
            n191 = Select(t=T12."Enabled" ("Disabled"), s=w277, f=T12."Disabled and Grayed Out" ("Disabled")) -> (s? t:f=w269:T12)
            n192 = local write "ProfInfo"(w281) -> ()
            n193 = local write "Process Found"(w277) -> ()
            n194 = local write "Identification"(w282) -> ()
            n195 = property on="ButtonTest" class="Bool (strict)"("DisabledEnum"=w269) -> (error out=w272:errorcluster)  [unwired: 2 in, 1 out]
            n196 = property on="ButtonResults" class="Bool (strict)"(error in=w272, "DisabledEnum"=w269) -> (error out=w270:errorcluster)  [unwired: 1 in, 1 out]
            n197 = local read "PrevTabState"() -> (w273:i32)
            n198 = property on="ButtonGoToTest" class="Bool (strict)"(error in=w270, "DisabledEnum"=w269) -> (error out=w271:errorcluster)  [unwired: 1 in, 1 out]
            n199 = case shown="True" w277 {
              selector: w277 -> [_ w285]
              tunnel: w273 -> [_ w286]
              frame False {
              }
              frame True {
                n200 = case shown="Default" w286 {
                  tunnel: w285 -> [w287 w288]
                  frame Default {
                    n201 = property on="ButtonGoToTest" class="Bool (strict)"("Val(Sgnl)"=w287) -> ()  [unwired: 2 in, 2 out]
                  }
                  frame 2 {
                    n202 = property on="ButtonGoToResults" class="Bool (strict)"("Val(Sgnl)"=w288) -> ()  [unwired: 2 in, 2 out]
                  }
                }
              }
            }
            n203 = property on="ButtonGoToResults" class="Bool (strict)"(error in=w271, "DisabledEnum"=w269) -> ()  [unwired: 1 in, 2 out]
          }
          event "ProcTree": event #0x1e {
            n204 = event-data() -> ("CtlRef"=w292:refnum<vi>, "Tag"=w290:string)  [unwired: 1 in]
            n205 = call "ProdaNG.Tree.Proc.GetTag.vi"("Tree"=w292, "Tag"=w290) -> ("parent"=w289:bool, "Identification"=w291:T7)  [unwired: 5 in, 3 out]
            n206 = case shown="True" w289 {
              tunnel: w296 -> [w298 w307]
              tunnel: w295 -> [w299 w306]
              tunnel: [w298 w305] -> w294
              tunnel: [w299 w304] -> w293
              tunnel: w291 -> [_ w302]
              tunnel: w290 -> [_ w300]
              frame False {
              }
              frame True {
                n207 = Unbundle By Name(w302) -> ("WP_ID"=w301:i32)
                n208 = control-ref of="ProcTree"() -> (w303:refnum<vi>)
                n209 = call "ProdaNG.WabcoPartProcesses.Get.vi"("error in (no error)"=w307, "WabcoPartId"=w301, "dbHandleIn"=w306) -> ("error out"=w310:errorcluster, "Proc"=w308:T20[], "dbHandle"=w309:i32)  [unwired: 6 in]
                n210 = Empty Array?(array=w308) -> (empty?=w311:bool)
                n211 = case shown="False" w311 {
                  tunnel: w310 -> [w313 w335]
                  tunnel: w309 -> [w319 w336]
                  tunnel: [w318 w336] -> w304
                  tunnel: [w317 w334] -> w305
                  tunnel: w308 -> [w320 _]
                  tunnel: w303 -> [w315 w333]
                  tunnel: w301 -> [w316 _]
                  tunnel: w300 -> [w314 w332]
                  frame False {
                    n212 = call "ProdaNG.Tree.WabcoPart.Clear.vi"("Tree"=w315, "error in (no error)"=w313, "Tag"=w314) -> ("error out"=w312:errorcluster)  [unwired: 8 in]
                    n213 = for {
                      tunnel: w319 -> [w331]
                      tunnel: [w324] -> w318
                      tunnel: w320 -> [w323] mode=indexing
                      shift-right: [w325] -> w317
                      shift-left: w312 -> [w329]
                      tunnel: w315 -> [w330]
                      tunnel: w316 -> [w321]
                      n214 = call "ProdaNG.Tree.Process.Add.vi"("Tree"=w330, "error in (no error)"=w329, "WabcoPartId"=w321, "ProcessStep"=w323) -> ("error out"=w328:errorcluster)  [unwired: 7 in]
                      n215 = Unbundle By Name(w323) -> ("i_id"=w322:i32)
                      n216 = call "ProdaNG.ProcessSteps.Get.vi"("error in (no error)"=w328, "processId"=w322, "dbHandleIn"=w331) -> ("error out"=w326:errorcluster, "ProcSteps"=w327:T22[], "dbHandle"=w324:i32)  [unwired: 6 in]
                      n217 = call "ProdaNG.Tree.ProcessSteps.Add.vi"("WabcoPartId"=w321, "Tree"=w330, "error in (no error)"=w326, "ProcId"=w322, "ProcSteps in"=w327) -> ("error out"=w325:errorcluster)  [unwired: 5 in, 1 out]
                    }
                  }
                  frame True {
                    n218 = call "ProdaNG.Tree.WabcoPart.Clear.vi"("Tree"=w333, "error in (no error)"=w335, "Tag"=w332) -> ("error out"=w334:errorcluster)  [unwired: 8 in]
                  }
                }
              }
            }
          }
          event "ButtonGoToTest": Value Change {
            w345 = T12."Disabled and Grayed Out" ("Disabled")
            n219 = event-data() -> ()  [unwired: 1 in, 1 out]
            n220 = property on="ButtonGoToTest" class="Bool (strict)"("Value"=FALSE ("ButtonGoToTest")) -> ()  [unwired: 2 in, 2 out]
            n221 = local read "ProfInfo"() -> (w348:string[])
            n222 = property on="ButtonTest" class="Bool (strict)"("Val(Sgnl)"=TRUE ("Value (Signaling)")) -> (error out=w339:errorcluster)  [unwired: 2 in, 1 out]
            n223 = Array To Spreadsheet String(delimiter (Tab)=" | ", array=w348, 3:"%s" ("format string")) -> (spreadsheet string=w342:string)
            n224 = call <vilib>:"Trim Whitespace.vi"("string"=w342) -> ("trimmed string"=→"Status":string)  [unwired: 1 in]
            n225 = property on="ButtonRefreshTestTree" class="Bool (strict)"(error in=w339, "Val(Sgnl)"=TRUE ("Value (Signaling)")) -> ()  [unwired: 1 in, 2 out]
            n226 = local write "SelectedFile"(path "") -> ()
            n227 = local write "FileInUse"("") -> ()
            n228 = property on="ButtonExportFile" class="Bool (strict)"("DisabledEnum"=w345) -> ()  [unwired: 2 in, 2 out]
            n229 = local write "FileContent"(T4 {"PP"=[], "TS"=[]} ("Seq")) -> ()
            n230 = property on="ButtonCloseFile" class="Bool"("DisabledEnum"=w345) -> ()  [unwired: 2 in, 2 out]
          }
          event "ButtonGoToResults": Value Change {
            n231 = event-data() -> ()  [unwired: 1 in, 1 out]
            n232 = property on="ButtonGoToResults" class="Bool (strict)"("Value"=FALSE ("ButtonGoToResults")) -> ()  [unwired: 2 in, 2 out]
            n233 = local read "ProfInfo"() -> (w360:string[])
            n234 = property on="ButtonResults" class="Bool (strict)"("Val(Sgnl)"=TRUE ("Value (Signaling)")) -> (error out=w355:errorcluster)  [unwired: 2 in, 1 out]
            n235 = Array To Spreadsheet String(delimiter (Tab)=" | ", array=w360, 3:"%s" ("format string")) -> (spreadsheet string=w357:string)
            n236 = call <vilib>:"Trim Whitespace.vi"("string"=w357) -> ("trimmed string"=w354:string)  [unwired: 1 in]
            n237 = property on="ButtonRefreshResultTree" class="Bool (strict)"(error in=w355, "Val(Sgnl)"=TRUE ("Value (Signaling)")) -> ()  [unwired: 1 in, 2 out]
            n238 = local write "Status"(w354) -> ()
          }
          event "ButtonRefreshTestTree": Value Change {
            n239 = event-data() -> ()  [unwired: 1 in, 1 out]
            n240 = property on="TestTree" class="Tree (strict)"() -> (error out=w367:errorcluster, "Value"=w369:string[], "TopLeft"=w368:T15)  [unwired: 2 in, 1 out]
            n241 = stacked-sequence {
              tunnel: [_ _ w393 _] -> w372
              tunnel: w370 -> [_ _ w390 _]
              tunnel: w366 -> [_ _ w392 _]
              tunnel: [_ _ w391 _] -> w365
              tunnel: w369 -> [_ _ _ w416]
              tunnel: w368 -> [_ _ _ w415]
              tunnel: w367 -> [_ _ _ w414]
              tunnel: [_ _ _ w413] -> _
              frame #0 {
                w373 = TRUE ("Value (Signaling)")
                n242 = property on="ButtonRefreshTestTree" class="Bool (strict)"("Value"=w373) -> ()  [unwired: 2 in, 2 out]
                n243 = property on="Progress" class="Bool (strict)"("Visible"=w373) -> ()  [unwired: 2 in, 2 out]
                n244 = property on="Hider" class="Bool (strict)"("Visible"=w373) -> ()  [unwired: 2 in, 2 out]
              }
              frame #1 {
                n245 = local read "FPref"() -> (w374:refnum<vi>)
                n246 = property class="Pnl"(reference=w374, "DeferPanUpdts"=TRUE ("Defer Panel Updates")) -> ()  [unwired: 1 in, 2 out]
              }
              frame #2 {
                n247 = local read "Identification"() -> (w388:T7)
                n248 = local read "FileContent"() -> (w378:T4)
                n249 = control-ref of="TestTree"() -> (w389:refnum<vi>)
                n250 = call "ProdaNG.Tree.Test.Update.vi"("Identification"=w388, "FileContent"=w378, "TreeControl in"=w389, "error in (no error)"=w392, "TreeViewMode (All)"="TestTreeView", "dbHandle in"=w390) -> ("error out"=w391:errorcluster, "#changes"=w380:i32, "Number of Rows"=w382:i32, "dbHandle out"=w393:i32)  [unwired: 2 in]
                n251 = Unbundle By Name(w378) -> ("TS"=w377:T6[])
                n252 = Greater Than 0?(x=w382) -> (x > 0?=w386:bool)
                n253 = Empty Array?(array=w377) -> (empty?=w376:bool)
                n254 = Select(t=T12."Enabled" ("Disabled"), s=w386, f=T12."Disabled and Grayed Out" ("Disabled")) -> (s? t:f=w383:T12)
                n255 = property on="ButtonUnreleaseAll" class="Bool"("DisabledEnum"=w383) -> ()  [unwired: 2 in, 2 out]
                n256 = case shown="True" w376 {
                  tunnel: [w396 "No file selected"] -> w381
                  tunnel: w380 -> [w395 _]
                  tunnel: [w394 u32 13816530] -> w379
                  frame False {
                    n257 = case shown="2.." w395 {
                      selector: w395 -> [_ w400 w404]
                      tunnel: ["No changes" w402 w406] -> w396
                      tunnel: [u32 13816530 u32 16744576 u32 16744576] -> w394
                      frame Default {
                      }
                      frame 1 {
                        n258 = Format Into String(format string="%d change", w400) -> (resulting string=w402:string)  [unwired: 2 in, 1 out]
                      }
                      frame 2.. {
                        n259 = Format Into String(format string="%d changes", w404) -> (resulting string=w406:string)  [unwired: 2 in, 1 out]
                      }
                    }
                  }
                  frame True {
                  }
                }
                n260 = property on="ButtonDeleteAll" class="Bool"("DisabledEnum"=w383) -> ()  [unwired: 2 in, 2 out]
                n261 = property on="FileInUse" class="Str"("Caption.Text"=w381, "Text.BGColor"=w379) -> ()  [unwired: 2 in, 2 out]
                n262 = property on="ButtonReleaseAll" class="Bool"("DisabledEnum"=w383) -> ()  [unwired: 2 in, 2 out]
              }
              frame #3 {
                w409 = FALSE ("Value (Signaling)")
                n263 = property on="TestTree" class="Tree (strict)"(error in=w414, "Val(Sgnl)"=w416, "TopLeft"=w415) -> (error out=w413:errorcluster)  [unwired: 1 in, 1 out]
                n264 = property on="ButtonRefreshTestTree" class="Bool (strict)"("Value"=w409) -> ()  [unwired: 2 in, 2 out]
                n265 = local read "FPref"() -> (w411:refnum<vi>)
                n266 = property class="Pnl"(reference=w411, "DeferPanUpdts"=FALSE ("Defer Panel Updates")) -> ()  [unwired: 1 in, 2 out]
                n267 = property on="Progress" class="Bool (strict)"("Visible"=w409) -> ()  [unwired: 2 in, 2 out]
                n268 = property on="Hider" class="Bool (strict)"("Visible"=w409) -> ()  [unwired: 2 in, 2 out]
                n269 = local write "TestTree.OpenCloseAll"(TRUE ("TestTree.OpenCloseAll")) -> ()
              }
            }
          }
          event "TestTree": Value Change {
            n270 = event-data() -> ("CtlRef"=w429:refnum<vi>)  [unwired: 1 in]
            n271 = call "ProdaNG.Tree.Release.Get.vi"("TestStepsTree"=w429, "error in (no error)"=w446, "Release"=TRUE) -> ("error out"=w438:errorcluster, "Elements to release"=w444:T23[])  [unwired: 7 in]
            n272 = call "ProdaNG.Tree.Release.Get.vi"("TestStepsTree"=w429, "error in (no error)"=w438, "Release"=FALSE) -> ("error out"=w431:errorcluster, "Elements to release"=w434:T23[])  [unwired: 7 in]
            n273 = call "ProdaNG.Tree.Selection.GetAll.vi"("TestStepsTree"=w429, "error in (no error)"=w431) -> ("error out"=w430:errorcluster, "Selected elements"=w423:T23[])  [unwired: 7 in, 1 out]
            n274 = Array Size(array=w423) -> (size(s)=w422:i32)
            n275 = Empty Array?(array=w444) -> (empty?=w443:bool)
            n276 = Empty Array?(array=w434) -> (empty?=w435:bool)
            n277 = Empty Array?(array=w423) -> (empty?=w428:bool)
            n278 = Greater?(x=w422, y=1) -> (0:w417:bool)
            n279 = Select(t=2 ("Disabled"), s=w443, f=0 ("Disabled")) -> (s? t:f=w440:i32)
            n280 = Select(t=2 ("Disabled"), s=w435, f=0 ("Disabled")) -> (s? t:f=w433:i32)
            n281 = Select(t=2 ("Disabled"), s=w428, f=0 ("Disabled")) -> (s? t:f=w424:i32)
            n282 = Select(t=2 ("Disabled"), s=w417, f=0 ("Disabled")) -> (s? t:f=w420:i32)
            n283 = property on="ButtonRelease" class="Bool"("DisabledEnum"=w440) -> ()  [unwired: 2 in, 2 out]
            n284 = property on="ButtonUnrelease" class="Bool"("DisabledEnum"=w433) -> ()  [unwired: 2 in, 2 out]
            n285 = property on="ButtonDelete" class="Bool"("DisabledEnum"=w424) -> (error out=w425:errorcluster)  [unwired: 2 in, 1 out]
            n286 = property on="ButtonAdd" class="Bool"("DisabledEnum"=w420) -> ()  [unwired: 2 in, 2 out]
            n287 = property on="ButtonEdit" class="Bool"(error in=w425, "DisabledEnum"=w424) -> ()  [unwired: 1 in, 2 out]
          }
          event "TestTree.OpenCloseAll": Value Change {
            w454 = 0 ("Active Item:Row Number")
            n288 = event-data() -> ()  [unwired: 1 in, 1 out]
            n289 = invoke on="TestTree" class="Tree (strict)" method="Open/Close.Open/Close All"("Open"="TestTree.OpenCloseAll") -> (error out=w451:errorcluster)  [unwired: 3 in, 3 out]
            n290 = property on="ResultsTree" class="Tree (strict)"(error in=w451, "Active Item Row Number"=w454, "ActiveColNum"=w454) -> (error out=w450:errorcluster, "Active Item Tag"=w453:string)  [unwired: 1 in, 1 out]
            n291 = Bundle By Name(cluster=T15 {"Node"="", "Column"=0} ("Top Left Visible Cell"), "Node"=w453) -> (w449:T15)
            n292 = property on="ResultsTree" class="Tree (strict)"(error in=w450, "TopLeft"=w449) -> (error out=w448:errorcluster)  [unwired: 1 in, 1 out]
            n293 = Unbundle(w448) -> ()  [unwired: 3 out]
          }
          event "ButtonRelease": Value Change {
            w463 = TRUE ("Release")
            n294 = event-data() -> ()  [unwired: 1 in, 1 out]
            n295 = control-ref of="TestTree"() -> (w464:refnum<vi>)
            n296 = call "ProdaNG.Tree.Release.Get.vi"("TestStepsTree"=w464, "error in (no error)"=w465, "Release"=w463) -> ("error out"=w460:errorcluster, "Elements to release"=w462:T23[])  [unwired: 7 in]
            n297 = Empty Array?(array=w462) -> (empty?=w461:bool)
            n298 = case shown="False" w461 {
              tunnel: w468 -> [w478 w502]
              tunnel: [w477 w501] -> w467
              tunnel: [w476 w502] -> w466
              tunnel: w460 -> [w475 w501]
              tunnel: w464 -> [w474 _]
              tunnel: w463 -> [w473 _]
              tunnel: w462 -> [w472 _]
              tunnel: w459 -> [w469 _]
              frame False {
                n299 = call "ProdaNG.Configurator.Popup.Release.vi"("Release"=w473, "Elements to release/unrelease"=w472) -> ("Reason out"=w471:string, "OK?"=w470:bool)  [unwired: 8 in]
                n300 = case shown="\"ProcessFound\"" w469 {
                  tunnel: w478 -> [w480 w489]
                  tunnel: [w479 w488] -> w477
                  tunnel: [w480 w487] -> w476
                  tunnel: w475 -> [w479 w486]
                  tunnel: w474 -> [_ w485]
                  tunnel: w473 -> [_ w484]
                  tunnel: w472 -> [_ w483]
                  tunnel: w471 -> [_ w482]
                  tunnel: w470 -> [_ w481]
                  frame Default {
                  }
                  frame "ProcessFound" {
                    n301 = case shown="True" w481 {
                      tunnel: w489 -> [w491 w500]
                      tunnel: [w490 w499] -> w488
                      tunnel: [w491 w498] -> w487
                      tunnel: w486 -> [w490 w497]
                      tunnel: w485 -> [_ w496]
                      tunnel: w483 -> [_ w495]
                      tunnel: w484 -> [_ w494]
                      tunnel: w482 -> [_ w492]
                      frame False {
                      }
                      frame True {
                        n302 = property on="ButtonRefreshTestTree" class="Bool (strict)"("Val(Sgnl)"=TRUE ("Value (Signaling)")) -> ()  [unwired: 2 in, 2 out]
                        n303 = call "ProdaNG.Tree.Release.vi"("comment"=w492, "TestStepsTree"=w496, "error in (no error)"=w497, "Release"=w494, "Elements to release/unrelease"=w495, "dbHandleIn"=w500) -> ("error out"=w499:errorcluster, "dbHandle"=w498:i32)  [unwired: 4 in]
                      }
                    }
                  }
                }
              }
              frame True {
              }
            }
          }
          event "ButtonReleaseAll": Value Change {
            w507 = TRUE ("Release")
            n304 = event-data() -> ()  [unwired: 1 in, 1 out]
            n305 = control-ref of="TestTree"() -> (w508:refnum<vi>)
            n306 = call "ProdaNG.Tree.Release.GetAll.vi"("TestStepsTree"=w508, "error in (no error)"=w509, "Release"=w507) -> ("error out"=w504:errorcluster, "Elements to release"=w506:T23[])  [unwired: 7 in]
            n307 = Empty Array?(array=w506) -> (empty?=w505:bool)
            n308 = case shown="False" w505 {
              tunnel: w512 -> [w522 w546]
              tunnel: [w521 w545] -> w511
              tunnel: [w520 w546] -> w510
              tunnel: w504 -> [w519 w545]
              tunnel: w508 -> [w518 _]
              tunnel: w507 -> [w517 _]
              tunnel: w506 -> [w516 _]
              tunnel: w503 -> [w513 _]
              frame False {
                n309 = call "ProdaNG.Configurator.Popup.Release.vi"("Release"=w517, "Elements to release/unrelease"=w516) -> ("Reason out"=w515:string, "OK?"=w514:bool)  [unwired: 8 in]
                n310 = case shown="\"ProcessFound\"" w513 {
                  tunnel: w522 -> [w524 w533]
                  tunnel: [w523 w532] -> w521
                  tunnel: [w524 w531] -> w520
                  tunnel: w519 -> [w523 w530]
                  tunnel: w518 -> [_ w529]
                  tunnel: w517 -> [_ w528]
                  tunnel: w516 -> [_ w527]
                  tunnel: w515 -> [_ w526]
                  tunnel: w514 -> [_ w525]
                  frame Default {
                  }
                  frame "ProcessFound" {
                    n311 = case shown="True" w525 {
                      tunnel: w533 -> [w535 w544]
                      tunnel: [w534 w543] -> w532
                      tunnel: [w535 w542] -> w531
                      tunnel: w530 -> [w534 w541]
                      tunnel: w529 -> [_ w540]
                      tunnel: w527 -> [_ w539]
                      tunnel: w528 -> [_ w538]
                      tunnel: w526 -> [_ w536]
                      frame False {
                      }
                      frame True {
                        n312 = property on="ButtonRefreshTestTree" class="Bool (strict)"("Val(Sgnl)"=TRUE ("Value (Signaling)")) -> ()  [unwired: 2 in, 2 out]
                        n313 = call "ProdaNG.Tree.Release.vi"("comment"=w536, "TestStepsTree"=w540, "error in (no error)"=w541, "Release"=w538, "Elements to release/unrelease"=w539, "dbHandleIn"=w544) -> ("error out"=w543:errorcluster, "dbHandle"=w542:i32)  [unwired: 4 in]
                      }
                    }
                  }
                }
              }
              frame True {
              }
            }
          }
          event "ButtonUnrelease": Value Change {
            w551 = FALSE ("Release")
            n314 = event-data() -> ()  [unwired: 1 in, 1 out]
            n315 = control-ref of="TestTree"() -> (w552:refnum<vi>)
            n316 = call "ProdaNG.Tree.Release.Get.vi"("TestStepsTree"=w552, "error in (no error)"=w553, "Release"=w551) -> ("error out"=w548:errorcluster, "Elements to release"=w550:T23[])  [unwired: 7 in]
            n317 = Empty Array?(array=w550) -> (empty?=w549:bool)
            n318 = case shown="False" w549 {
              tunnel: w556 -> [w566 w590]
              tunnel: [w565 w589] -> w555
              tunnel: [w564 w590] -> w554
              tunnel: w548 -> [w563 w589]
              tunnel: w552 -> [w562 _]
              tunnel: w551 -> [w561 _]
              tunnel: w550 -> [w560 _]
              tunnel: w547 -> [w557 _]
              frame False {
                n319 = call "ProdaNG.Configurator.Popup.Release.vi"("Release"=w561, "Elements to release/unrelease"=w560) -> ("Reason out"=w559:string, "OK?"=w558:bool)  [unwired: 8 in]
                n320 = case shown="\"ProcessFound\"" w557 {
                  tunnel: w566 -> [w568 w577]
                  tunnel: [w567 w576] -> w565
                  tunnel: [w568 w575] -> w564
                  tunnel: w563 -> [w567 w574]
                  tunnel: w562 -> [_ w573]
                  tunnel: w561 -> [_ w572]
                  tunnel: w560 -> [_ w571]
                  tunnel: w559 -> [_ w570]
                  tunnel: w558 -> [_ w569]
                  frame Default {
                  }
                  frame "ProcessFound" {
                    n321 = case shown="True" w569 {
                      tunnel: w577 -> [w579 w588]
                      tunnel: [w578 w587] -> w576
                      tunnel: [w579 w586] -> w575
                      tunnel: w574 -> [w578 w585]
                      tunnel: w573 -> [_ w584]
                      tunnel: w571 -> [_ w583]
                      tunnel: w572 -> [_ w582]
                      tunnel: w570 -> [_ w580]
                      frame False {
                      }
                      frame True {
                        n322 = property on="ButtonRefreshTestTree" class="Bool (strict)"("Val(Sgnl)"=TRUE ("Value (Signaling)")) -> ()  [unwired: 2 in, 2 out]
                        n323 = call "ProdaNG.Tree.Release.vi"("comment"=w580, "TestStepsTree"=w584, "error in (no error)"=w585, "Release"=w582, "Elements to release/unrelease"=w583, "dbHandleIn"=w588) -> ("error out"=w587:errorcluster, "dbHandle"=w586:i32)  [unwired: 4 in]
                      }
                    }
                  }
                }
              }
              frame True {
              }
            }
          }
          event "ButtonUnreleaseAll": Value Change {
            w595 = FALSE ("Release")
            n324 = event-data() -> ()  [unwired: 1 in, 1 out]
            n325 = control-ref of="TestTree"() -> (w596:refnum<vi>)
            n326 = call "ProdaNG.Tree.Release.GetAll.vi"("TestStepsTree"=w596, "error in (no error)"=w597, "Release"=w595) -> ("error out"=w592:errorcluster, "Elements to release"=w594:T23[])  [unwired: 7 in]
            n327 = Empty Array?(array=w594) -> (empty?=w593:bool)
            n328 = case shown="False" w593 {
              tunnel: w600 -> [w610 w634]
              tunnel: [w609 w633] -> w599
              tunnel: [w608 w634] -> w598
              tunnel: w592 -> [w607 w633]
              tunnel: w596 -> [w606 _]
              tunnel: w595 -> [w605 _]
              tunnel: w594 -> [w604 _]
              tunnel: w591 -> [w601 _]
              frame False {
                n329 = call "ProdaNG.Configurator.Popup.Release.vi"("Release"=w605, "Elements to release/unrelease"=w604) -> ("Reason out"=w603:string, "OK?"=w602:bool)  [unwired: 8 in]
                n330 = case shown="\"ProcessFound\"" w601 {
                  tunnel: w610 -> [w612 w621]
                  tunnel: [w611 w620] -> w609
                  tunnel: [w612 w619] -> w608
                  tunnel: w607 -> [w611 w618]
                  tunnel: w606 -> [_ w617]
                  tunnel: w605 -> [_ w616]
                  tunnel: w604 -> [_ w615]
                  tunnel: w603 -> [_ w614]
                  tunnel: w602 -> [_ w613]
                  frame Default {
                  }
                  frame "ProcessFound" {
                    n331 = case shown="True" w613 {
                      tunnel: w621 -> [w623 w632]
                      tunnel: [w622 w631] -> w620
                      tunnel: [w623 w630] -> w619
                      tunnel: w618 -> [w622 w629]
                      tunnel: w617 -> [_ w628]
                      tunnel: w615 -> [_ w627]
                      tunnel: w616 -> [_ w626]
                      tunnel: w614 -> [_ w624]
                      frame False {
                      }
                      frame True {
                        n332 = property on="ButtonRefreshTestTree" class="Bool (strict)"("Val(Sgnl)"=TRUE ("Value (Signaling)")) -> ()  [unwired: 2 in, 2 out]
                        n333 = call "ProdaNG.Tree.Release.vi"("comment"=w624, "TestStepsTree"=w628, "error in (no error)"=w629, "Release"=w626, "Elements to release/unrelease"=w627, "dbHandleIn"=w632) -> ("error out"=w631:errorcluster, "dbHandle"=w630:i32)  [unwired: 4 in]
                      }
                    }
                  }
                }
              }
              frame True {
              }
            }
          }
          event "ButtonAdd": Value Change {
            n334 = event-data() -> ()  [unwired: 1 in, 1 out]
            n335 = control-ref of="TestTree"() -> (w652:refnum<vi>)
            n336 = call "ProdaNG.Units.Get.vi"("error in (no error)"=w642, "dbHandleIn"=w641) -> ("error out"=w640:errorcluster, "units simple"=w638:T25[], "dbHandle"=w639:i32)  [unwired: 6 in, 1 out]
            n337 = call "ProdaNG.Tree.Selection.GetTS.vi"("TestStepsTree"=w652, "error in (no error)"=w640) -> ("error out"=w650:errorcluster, "Selected Element"=w636:T5, "LastTS"=w651:T23, "Eleemnt Type"=w635:T24)  [unwired: 6 in]
            n338 = local read "Identification"() -> (w643:T7)
            n339 = call "ProdaNG.Configurator.Popup.Add.vi"("units simple"=w638, "Eleemnt Type"=w635, "Selected Element"=w636, "LastTS"=w651) -> ("Selected elements value out"=w645:T5, "Selected element out"=w637:T23, "Reason out"=w644:string, "OK?"=w646:bool)  [unwired: 4 in]
            n340 = case shown="\"ProcessFound\"" w647 {
              tunnel: w639 -> [w653 w664]
              tunnel: [w654 w663] -> w649
              tunnel: [w653 w662] -> w648
              tunnel: w650 -> [w654 w661]
              tunnel: w652 -> [_ w660]
              tunnel: w637 -> [_ w659]
              tunnel: w646 -> [_ w658]
              tunnel: w645 -> [_ w657]
              tunnel: w644 -> [_ w656]
              tunnel: w643 -> [_ w655]
              frame Default {
              }
              frame "ProcessFound" {
                n341 = case shown="True" w658 {
                  tunnel: w664 -> [w666 w676]
                  tunnel: [w665 w675] -> w663
                  tunnel: [w666 w674] -> w662
                  tunnel: w661 -> [w665 w673]
                  tunnel: w660 -> [_ w672]
                  tunnel: w659 -> [_ w671]
                  tunnel: w657 -> [_ w668]
                  tunnel: w656 -> [_ w669]
                  tunnel: w655 -> [_ w667]
                  frame False {
                  }
                  frame True {
                    n342 = property on="ButtonRefreshTestTree" class="Bool (strict)"("Val(Sgnl)"=TRUE ("Value (Signaling)")) -> ()  [unwired: 2 in, 2 out]
                    n343 = call "ProdaNG.Tree.Add.vi"("Identification"=w667, "reason"=w669, "TestStepsTree"=w672, "error in (no error)"=w673, "Element values"=w668, "Element to add"=w671, "dbHandleIn"=w676) -> ("error out"=w675:errorcluster, "dbHandle"=w674:i32)  [unwired: 3 in]
                  }
                }
              }
            }
          }
          event "ButtonEdit": Value Change; "TestTree": Double Click {
            n344 = event-data() -> ()  [unwired: 1 in, 1 out]
            n345 = control-ref of="TestTree"() -> (w689:refnum<vi>)
            n346 = call "ProdaNG.Units.Get.vi"("error in (no error)"=w681, "dbHandleIn"=w678) -> ("error out"=w680:errorcluster, "units simple"=w677:T25[], "dbHandle"=w679:i32)  [unwired: 6 in, 1 out]
            n347 = call "ProdaNG.Tree.Selection.GetAll.vi"("TestStepsTree"=w689, "error in (no error)"=w680) -> ("error out"=w686:errorcluster, "Selected elements values"=w682:T5[], "Selected elements"=w688:T23[])  [unwired: 7 in]
            n348 = Empty Array?(array=w688) -> (empty?=w687:bool)
            n349 = case shown="False" w687 {
              tunnel: w679 -> [w701 w725]
              tunnel: [w700 w724] -> w685
              tunnel: [w699 w725] -> w684
              tunnel: w686 -> [w698 w724]
              tunnel: w689 -> [w697 _]
              tunnel: w688 -> [w696 _]
              tunnel: w683 -> [w694 _]
              tunnel: w682 -> [w693 _]
              tunnel: w677 -> [w690 _]
              frame False {
                n350 = call "ProdaNG.Configurator.Popup.Edit.vi"("units simple"=w690, "Selected elements values"=w693, "Elements to edit"=w696) -> ("Selected elements values out"=w692:T5[], "Reason out"=w691:string, "OK?"=w695:bool)  [unwired: 6 in]
                n351 = case shown="\"ProcessFound\"" w694 {
                  tunnel: w701 -> [w702 w712]
                  tunnel: [w703 w711] -> w700
                  tunnel: [w702 w710] -> w699
                  tunnel: w698 -> [w703 w709]
                  tunnel: w697 -> [_ w708]
                  tunnel: w696 -> [_ w707]
                  tunnel: w695 -> [_ w706]
                  tunnel: w692 -> [_ w705]
                  tunnel: w691 -> [_ w704]
                  frame Default {
                  }
                  frame "ProcessFound" {
                    n352 = case shown="True" w706 {
                      tunnel: w712 -> [w714 w723]
                      tunnel: [w713 w722] -> w711
                      tunnel: [w714 w721] -> w710
                      tunnel: w709 -> [w713 w720]
                      tunnel: w708 -> [_ w719]
                      tunnel: w707 -> [_ w718]
                      tunnel: w705 -> [_ w716]
                      tunnel: w704 -> [_ w717]
                      frame False {
                      }
                      frame True {
                        n353 = property on="ButtonRefreshTestTree" class="Bool (strict)"("Val(Sgnl)"=TRUE ("Value (Signaling)")) -> ()  [unwired: 2 in, 2 out]
                        n354 = call "ProdaNG.Tree.Edit.vi"("reason"=w717, "TestStepsTree"=w719, "error in (no error)"=w720, "Selected elements values"=w716, "Selected elements"=w718, "dbHandleIn"=w723) -> ("error out"=w722:errorcluster, "dbHandle"=w721:i32)  [unwired: 4 in]
                      }
                    }
                  }
                }
              }
              frame True {
              }
            }
          }
          event "ButtonDelete": Value Change {
            n355 = event-data() -> ()  [unwired: 1 in, 1 out]
            n356 = control-ref of="TestTree"() -> (w734:refnum<vi>)
            n357 = call "ProdaNG.Tree.Selection.GetAll.vi"("TestStepsTree"=w734, "error in (no error)"=w730) -> ("error out"=w731:errorcluster, "Selected elements"=w733:T23[])  [unwired: 7 in, 1 out]
            n358 = Empty Array?(array=w733) -> (empty?=w732:bool)
            n359 = case shown="False" w732 {
              tunnel: w729 -> [w742 w762]
              tunnel: [w741 w761] -> w728
              tunnel: [w740 w762] -> w727
              tunnel: w731 -> [w739 w761]
              tunnel: w734 -> [w738 _]
              tunnel: w733 -> [w737 _]
              tunnel: w726 -> [w735 _]
              frame False {
                n360 = call "ProdaNG.Configurator.Popup.Delete.vi"("Elements to delete"=w737) -> ("OK?"=w736:bool)  [unwired: 10 in]
                n361 = case shown="\"ProcessFound\"" w735 {
                  tunnel: w742 -> [w743 w751]
                  tunnel: [w744 w750] -> w741
                  tunnel: [w743 w749] -> w740
                  tunnel: w739 -> [w744 w748]
                  tunnel: w738 -> [_ w747]
                  tunnel: w737 -> [_ w746]
                  tunnel: w736 -> [_ w745]
                  frame Default {
                  }
                  frame "ProcessFound" {
                    n362 = case shown="True" w745 {
                      tunnel: w751 -> [w753 w760]
                      tunnel: [w752 w759] -> w750
                      tunnel: [w753 w758] -> w749
                      tunnel: w748 -> [w752 w757]
                      tunnel: w747 -> [_ w756]
                      tunnel: w746 -> [_ w755]
                      frame False {
                      }
                      frame True {
                        n363 = property on="ButtonRefreshTestTree" class="Bool (strict)"("Val(Sgnl)"=TRUE ("Value (Signaling)")) -> ()  [unwired: 2 in, 2 out]
                        n364 = call "ProdaNG.Tree.Delete.vi"("TestStepsTree"=w756, "error in (no error)"=w757, "Elements to delete"=w755, "dbHandleIn"=w760) -> ("error out"=w759:errorcluster, "dbHandle"=w758:i32)  [unwired: 6 in]
                      }
                    }
                  }
                }
              }
              frame True {
              }
            }
          }
          event "ButtonDeleteAll": Value Change {
            n365 = event-data() -> ()  [unwired: 1 in, 1 out]
            n366 = control-ref of="TestTree"() -> (w771:refnum<vi>)
            n367 = call "ProdaNG.Tree.GetAll.vi"("TestStepsTree"=w771, "error in (no error)"=w767) -> ("error out"=w768:errorcluster, "Selected elements"=w770:T23[])  [unwired: 7 in, 1 out]
            n368 = Empty Array?(array=w770) -> (empty?=w769:bool)
            n369 = case shown="False" w769 {
              tunnel: w766 -> [w779 w799]
              tunnel: [w778 w798] -> w765
              tunnel: [w777 w799] -> w764
              tunnel: w768 -> [w776 w798]
              tunnel: w771 -> [w775 _]
              tunnel: w770 -> [w774 _]
              tunnel: w763 -> [w772 _]
              frame False {
                n370 = call "ProdaNG.Configurator.Popup.Delete.vi"("Elements to delete"=w774) -> ("OK?"=w773:bool)  [unwired: 10 in]
                n371 = case shown="\"ProcessFound\"" w772 {
                  tunnel: w779 -> [w780 w788]
                  tunnel: [w781 w787] -> w778
                  tunnel: [w780 w786] -> w777
                  tunnel: w776 -> [w781 w785]
                  tunnel: w775 -> [_ w784]
                  tunnel: w774 -> [_ w783]
                  tunnel: w773 -> [_ w782]
                  frame Default {
                  }
                  frame "ProcessFound" {
                    n372 = case shown="True" w782 {
                      tunnel: w788 -> [w790 w797]
                      tunnel: [w789 w796] -> w787
                      tunnel: [w790 w795] -> w786
                      tunnel: w785 -> [w789 w794]
                      tunnel: w784 -> [_ w793]
                      tunnel: w783 -> [_ w792]
                      frame False {
                      }
                      frame True {
                        n373 = property on="ButtonRefreshTestTree" class="Bool (strict)"("Val(Sgnl)"=TRUE ("Value (Signaling)")) -> ()  [unwired: 2 in, 2 out]
                        n374 = call "ProdaNG.Tree.Delete.vi"("TestStepsTree"=w793, "error in (no error)"=w794, "Elements to delete"=w792, "dbHandleIn"=w797) -> ("error out"=w796:errorcluster, "dbHandle"=w795:i32)  [unwired: 6 in]
                      }
                    }
                  }
                }
              }
              frame True {
              }
            }
          }
          event "ButtonOpenFile": Value Change {
            n375 = event-data() -> ()  [unwired: 1 in, 1 out]
            n376 = local read "SelectedFile"() -> (w801:path)
            n377 = call "File exists.vi"("file path"=w801) -> ("exists?"=w802:bool)  [unwired: 4 in]
            n378 = case shown="True" w802 {
              tunnel: [w817 TRUE] -> w808
              tunnel: [w814 w820] -> w807
              tunnel: w806 -> [w812 w819]
              tunnel: [w811 w819] -> w804
              tunnel: w801 -> [_ w820]
              frame False {
                n379 = call "File Dialog2"("prompt"="Select seqeunce configuration flie...", "error in"=w812, "pattern (all files)"="*.ini") -> ("selected path"=w814:path, "exists"=w810:bool, "cancelled"=w815:bool, "error out"=w811:errorcluster)  [unwired: 9 in]
                n380 = Compound Arithmetic op=AND(w810, invert w815) -> (w817:bool)
              }
              frame True {
              }
            }
            n381 = case shown="True" w808 {
              tunnel: w804 -> [w822 w831]
              tunnel: w807 -> [_ w828]
              tunnel: [w821 w825] -> w805
              tunnel: w803 -> [_ w832]
              frame False {
                n382 = call <vilib>:"Clear Errors.vi"("error in (no error)"=w822) -> ("error out"=w821:errorcluster)  [unwired: 5 in, 1 out]
              }
              frame True {
                n383 = local read "SlotInUse"() -> (w823:i32)
                n384 = call "ProdaNG.Units.Get.vi"("error in (no error)"=w831, "dbHandleIn"=w832) -> ("error out"=w830:errorcluster, "units simple"=w829:T25[])  [unwired: 6 in, 2 out]
                n385 = call "ProdaNG.File.Read.vi"("Config"="Configuration", "error in (no error)"=w830, "units"=w829, "SeqFile Path"=w828, "SlotNo"=w823) -> ("error out"=w825:errorcluster, "Seq"=w826:T4)  [unwired: 4 in, 1 out]
                n386 = call <vilib>:"Get File Extension.vi"("file"=w828) -> ("filename without extension"=w827:string)  [unwired: 6 in, 4 out]
                n387 = case shown="No Error" w825 {
                  tunnel: w827 -> [w844 _]
                  tunnel: w826 -> [w839 _]
                  tunnel: w823 -> [w837 _]
                  frame No Error {
                    w847 = T12."Enabled" ("Disabled")
                    n388 = property on="ButtonRefreshTestTree" class="Bool (strict)"("Val(Sgnl)"=TRUE ("Value (Signaling)")) -> ()  [unwired: 2 in, 2 out]
                    n389 = Compound Arithmetic op=ADD(w837, 65 ("value")) -> (w846:i32)
                    n390 = Build Array(w846) -> (w843:i32[])
                    n391 = Greater Or Equal To 0?(x=w837) -> (x >= 0?=w836:bool)
                    n392 = property on="ButtonExportFile" class="Bool (strict)"("DisabledEnum"=w847) -> ()  [unwired: 2 in, 2 out]
                    n393 = Byte Array To String(unsigned byte array=w843) -> (string=w838:string)
                    n394 = Select(t=w838, s=w836, f="") -> (s? t:f=w834:string)
                    n395 = Format Into String(format string="%s %s", w844, w834) -> (resulting string=w841:string)  [unwired: 2 in, 1 out]
                    n396 = property on="ButtonCloseFile" class="Bool"("DisabledEnum"=w847) -> ()  [unwired: 2 in, 2 out]
                    n397 = call <vilib>:"Trim Whitespace.vi"("string"=w841) -> ("trimmed string"=→"FileInUse":string)  [unwired: 1 in]
                    n398 = property on="FileInUse" class="Str"("Text.BGColor"=u32 13816530) -> ()  [unwired: 2 in, 2 out]
                    "FileContent" <- w839
                  }
                  frame Error {
                  }
                }
                "SelectedFile" <- w828
              }
            }
            n399 = property on="ButtonOpenFile" class="Bool (strict)"("Value"=FALSE ("ButtonOpenFile")) -> ()  [unwired: 2 in, 2 out]
          }
          event "ButtonCloseFile": Value Change {
            w851 = T12."Disabled and Grayed Out" ("Disabled")
            n400 = event-data() -> ()  [unwired: 1 in, 1 out]
            n401 = property on="ButtonExportFile" class="Bool (strict)"("DisabledEnum"=w851) -> ()  [unwired: 2 in, 2 out]
            n402 = local write "FileContent"(T4 {"PP"=[], "TS"=[]} ("Seq")) -> ()
            n403 = local write "SelectedFile"(path "" ("SelectedFile")) -> ()
            n404 = local write "FileInUse"("") -> ()
            n405 = property on="ButtonCloseFile" class="Bool"("DisabledEnum"=w851) -> ()  [unwired: 2 in, 2 out]
            n406 = property on="ButtonRefreshTestTree" class="Bool (strict)"("Val(Sgnl)"=TRUE ("Value (Signaling)")) -> ()  [unwired: 2 in, 2 out]
          }
          event "ButtonExportFile": Value Change {
            n407 = event-data() -> ()  [unwired: 1 in, 1 out]
            n408 = Two Button Dialog(message="Data will be exported to production database!!!\n\n Do you want to continue?") -> (T button?=w858:bool)  [unwired: 2 in]
            n409 = case shown="True" w858 {
              tunnel: w862 -> [w865 w870]
              tunnel: w861 -> [w864 w869]
              tunnel: [w865 w868] -> w860
              tunnel: [w864 w867] -> w859
              frame False {
                n410 = property on="ButtonExportFile" class="Bool (strict)"("Value"=FALSE ("ButtonExportFile")) -> ()  [unwired: 2 in, 2 out]
              }
              frame True {
                n411 = stacked-sequence {
                  tunnel: w870 -> [_ w881 _]
                  tunnel: w869 -> [_ w880 _]
                  tunnel: [_ w876 _] -> w868
                  tunnel: [_ w875 _] -> w867
                  frame #0 {
                    w871 = TRUE ("Visible")
                    n412 = local read "FPref"() -> (w872:refnum<vi>)
                    n413 = property on="Hider" class="Bool (strict)"("Visible"=w871) -> ()  [unwired: 2 in, 2 out]
                    n414 = property on="Progress" class="Bool (strict)"("Visible"=w871) -> ()  [unwired: 2 in, 2 out]
                    n415 = property class="Pnl"(reference=w872, "DeferPanUpdts"=TRUE ("Defer Panel Updates")) -> ()  [unwired: 1 in, 2 out]
                  }
                  frame #1 {
                    n416 = local read "Identification"() -> (w874:T7)
                    n417 = local read "FileContent"() -> (w878:T4)
                    n418 = control-ref of="TestTree"() -> (w879:refnum<vi>)
                    n419 = call "ProdaNG.File.ExportToDB.vi"("Identification"=w874, "reason"="Exported by Proda Configurator", "TestStepsTree"=w879, "error in (no error)"=w880, "FileContent"=w878, "dbHandleIn"=w881) -> ("error out"=w875:errorcluster, "dbHandle"=w876:i32)  [unwired: 4 in]
                  }
                  frame #2 {
                    w882 = FALSE ("Visible")
                    n420 = local read "FPref"() -> (w885:refnum<vi>)
                    n421 = property on="ButtonExportFile" class="Bool (strict)"("Value"=FALSE ("ButtonExportFile")) -> ()  [unwired: 2 in, 2 out]
                    n422 = property on="Hider" class="Bool (strict)"("Visible"=w882) -> ()  [unwired: 2 in, 2 out]
                    n423 = property class="Pnl"(reference=w885, "DeferPanUpdts"=FALSE ("Defer Panel Updates")) -> ()  [unwired: 1 in, 2 out]
                    n424 = property on="Progress" class="Bool (strict)"("Visible"=w882) -> ()  [unwired: 2 in, 2 out]
                    n425 = property on="ButtonRefreshTestTree" class="Bool (strict)"("Val(Sgnl)"=TRUE ("Value (Signaling)")) -> ()  [unwired: 2 in, 2 out]
                  }
                }
              }
            }
          }
          event "ButtonSaveToFile": Value Change {
            n426 = event-data() -> ()  [unwired: 1 in, 1 out]
            n427 = local read "ProfInfo"() -> (w887:string[])
            n428 = local read "SelectedFile"() -> (w901:path)
            n429 = call "File exists.vi"("file path"=w901) -> ("exists?"=w902:bool)  [unwired: 4 in]
            n430 = Index Array(array=w887) -> (element=w895:string)  [unwired: 1 in]
            n431 = call <vilib>:"Space Constant.vi"() -> ("String"=w893:string)
            n432 = call "ProdaNG.Units.Get.vi"("error in (no error)"=w891, "dbHandleIn"=w892) -> ("error out"=w889:errorcluster, "units simple"=w888:T25[], "dbHandle"=w890:i32)  [unwired: 6 in, 1 out]
            n433 = Match Pattern(string=w895, regular expression=w893) -> (before substring=w894:string)  [unwired: 1 in, 3 out]
            n434 = Concatenate Strings(w894, ".ini" ("string")) -> (w897:string)
            n435 = case shown="False" w902 {
              tunnel: w901 -> [_ w914]
              tunnel: [w909 w914] -> w900
              tunnel: [w908 w912] -> w899
              tunnel: w897 -> [w905 _]
              tunnel: [w907 w916] -> w896
              tunnel: w889 -> [w906 w916]
              frame False {
                n436 = call "File Dialog"("prompt"="Select seqeunce configuration flie...", "default name"=w905, "error in"=w906, "pattern (all files)"="*.ini") -> ("selected path"=w909:path, "cancelled"=w908:bool, "error out"=w907:errorcluster)  [unwired: 8 in, 1 out]
              }
              frame True {
                n437 = Two Button Dialog(message="File will be overwritten. Do you want to continue?") -> (T button?=w913:bool)  [unwired: 2 in]
                n438 = Not(x=w913) -> (.not. x?=w912:bool)
              }
            }
            n439 = case shown="False" w899 {
              tunnel: w896 -> [w924 w927]
              tunnel: [w926 w927] -> w903
              tunnel: w900 -> [w919 _]
              tunnel: w888 -> [w918 _]
              tunnel: w887 -> [w917 _]
              frame False {
                n440 = call "ProdaNG.File.ExportToFile.vi"("error in (no error)"=w924) -> ("error out"=w923:errorcluster, "FileContent"=w922:T4)  [unwired: 9 in]
                n441 = local write "SelectedFile"(w919) -> ()
                n442 = local read "Configuration"() -> (w921:T8)
                n443 = local write "FileContent"(w922) -> ()
                n444 = property on="ButtonOpenFile" class="Bool (strict)"("Val(Sgnl)"=TRUE ("ButtonOpenFile")) -> ()  [unwired: 2 in, 2 out]
                n445 = local read "SlotInUse"() -> (w925:i32)
                n446 = call "ProdaNG.File.Write.vi"("ProfInfo"=w917, "Config"=w921, "SlotNo"=w925, "error in (no error)"=w923, "units"=w918, "Seq"=w922, "SeqFile Path"=w919) -> ("error out"=w926:errorcluster)  [unwired: 4 in]
              }
              frame True {
              }
            }
          }
          event "ButtonRefreshResultTree": Value Change {
            n447 = event-data() -> ()  [unwired: 1 in, 1 out]
            n448 = property on="ResultsTree" class="Tree (strict)"() -> (error out=w930:errorcluster, "Value"=w932:string[], "TopLeft"=w931:T15)  [unwired: 2 in, 1 out]
            n449 = stacked-sequence {
              tunnel: [_ _ _ w991 _] -> w935
              tunnel: w933 -> [_ _ _ w985 _]
              tunnel: w929 -> [_ _ _ w986 _]
              tunnel: [_ _ _ w989 _] -> w928
              tunnel: w932 -> [_ _ _ _ w1009]
              tunnel: w931 -> [_ _ _ _ w1008]
              tunnel: w930 -> [_ _ _ _ w1007]
              tunnel: [_ _ _ _ w1006] -> _
              frame #0 {
                w936 = TRUE ("Value (Signaling)")
                n450 = property on="ButtonRefreshResultTree" class="Bool (strict)"("Value"=w936) -> ()  [unwired: 2 in, 2 out]
                n451 = property on="Progress" class="Bool (strict)"("Visible"=w936) -> ()  [unwired: 2 in, 2 out]
                n452 = property on="Hider" class="Bool (strict)"("Visible"=w936) -> ()  [unwired: 2 in, 2 out]
              }
              frame #1 {
                n453 = local read "FPref"() -> (w937:refnum<vi>)
                n454 = property class="Pnl"(reference=w937, "DeferPanUpdts"=TRUE ("Defer Panel Updates")) -> ()  [unwired: 1 in, 2 out]
              }
              frame #2 {
                n455 = local read "DBtime"() -> (w941:timestamp)
                n456 = case shown="\"Custom\"" "ResultsSpan" {
                  tunnel: [w945 w949 w955 w960 w965 w970] -> w943
                  tunnel: w941 -> [_ w950 w955 w960 w965 w970]
                  tunnel: [w944 w946 w956 w961 w966 w971] -> w940
                  tunnel: "ResultsAmount" -> [_ w948 w954 w959 w964 w969]
                  frame "Custom" {
                    n457 = local read "Results.TimeFrom"() -> (w944:timestamp)
                    n458 = local read "Results.TimeTo"() -> (w945:timestamp)
                  }
                  frame "Shift(s)" {
                    n459 = call "GetShiftTime.vi"("Time"=w950) -> ("Shift End Time"=w949:timestamp)  [unwired: 7 in, 3 out]
                    n460 = Compound Arithmetic op=MULTIPLY(w948, 28800) -> (w947:i32)
                    n461 = Subtract(x=w949, y=w947) -> (x-y=w946:timestamp)
                  }
                  frame "Hour(s)" {
                    n462 = Compound Arithmetic op=MULTIPLY(w954, 3600) -> (w953:i32)
                    n463 = Subtract(x=w955, y=w953) -> (x-y=w956:timestamp)
                  }
                  frame "Day(s)" {
                    n464 = Compound Arithmetic op=MULTIPLY(w959, 86400) -> (w958:i32)
                    n465 = Subtract(x=w960, y=w958) -> (x-y=w961:timestamp)
                  }
                  frame "Week(s)" {
                    n466 = Compound Arithmetic op=MULTIPLY(w964, 604800) -> (w963:i32)
                    n467 = Subtract(x=w965, y=w963) -> (x-y=w966:timestamp)
                  }
                  frame "Month(s)" {
                    n468 = Compound Arithmetic op=MULTIPLY(w969, 2592000) -> (w968:i32)
                    n469 = Subtract(x=w970, y=w968) -> (x-y=w971:timestamp)
                  }
                }
                n470 = local write "Results.TimeFrom"(w940) -> ()
                n471 = local write "Results.TimeTo"(w943) -> ()
              }
              frame #3 {
                w982 = "%d.%m.%Y %H:%M:%S" ("time format string")
                n472 = local read "Identification"() -> (w992:T7)
                n473 = property on="ProductList" class="LstBox (strict)"(error in=w986) -> (error out=w993:errorcluster, "Item Names"=w995:string[], "Value"=w994:i32[])  [unwired: 1 in, 1 out]
                n474 = for {
                  tunnel: w995 -> [w1001]
                  tunnel: w994 -> [w1002] mode=indexing
                  tunnel: [w1000] -> w988 mode=indexing
                  n475 = Index Array(array=w1001, index=w1002) -> (element=w1000:string)
                }
                n476 = Unbundle By Name(w992) -> ("WP_ID"=w977:i32, "PS_ID"=w976:i32)
                n477 = Format Date/Time String(time format string (%c)=w982, seconds (now)="Results.TimeTo") -> (date/time string=w981:string)  [unwired: 1 in]
                n478 = Format Date/Time String(time format string (%c)=w982, seconds (now)="Results.TimeFrom") -> (date/time string=w980:string)  [unwired: 1 in]
                n479 = call "ProdaNG.Products.Get.vi"("Time To"=w981, "Time From"=w980, "error in (no error)"=w993, "proccessStepId (0: all)"=w976, "wabcoPartId"=w977, "dbHandleIn"=w985) -> ("error out"=w990:errorcluster, "Serials"=w978:string[], "Products"=w975:T1[], "dbHandle"=w991:i32)  [unwired: 2 in]
                "Products" <- w975
                n480 = Array Size(array=w975) -> (size(s)=w974:i32)
                n481 = Format Into String(format string="Products #%d" ("Caption.Text"), w974) -> (resulting string=w972:string)  [unwired: 2 in, 1 out]
                n482 = for {
                  tunnel: w978 -> [w999]
                  tunnel: w988 -> [w998] mode=indexing
                  tunnel: [w997] -> w987 mode=indexing if=w996
                  n483 = Search 1D Array(1D array=w999, element=w998) -> (index of element=w997:i32)  [unwired: 1 in]
                  n484 = Greater Or Equal To 0?(x=w997) -> (x >= 0?=w996:bool)
                }
                n485 = property on="ProductList" class="LstBox (strict)"("Caption.Text"=w972) -> ()  [unwired: 2 in, 2 out]
                n486 = property on="ProductList" class="LstBox (strict)"(error in=w990, "Item Names"=w978, "Val(Sgnl)"=w987, "Top Row"=0) -> (error out=w989:errorcluster)  [unwired: 1 in, 1 out]
              }
              frame #4 {
                w1003 = FALSE ("Value (Signaling)")
                n487 = property on="ResultsTree" class="Tree (strict)"(error in=w1007, "Val(Sgnl)"=w1009, "TopLeft"=w1008) -> (error out=w1006:errorcluster)  [unwired: 1 in, 1 out]
                n488 = property on="ButtonRefreshResultTree" class="Bool (strict)"("Value"=w1003) -> ()  [unwired: 2 in, 2 out]
                n489 = local read "FPref"() -> (w1004:refnum<vi>)
                n490 = property class="Pnl"(reference=w1004, "DeferPanUpdts"=FALSE ("Defer Panel Updates")) -> ()  [unwired: 1 in, 2 out]
                n491 = property on="Progress" class="Bool (strict)"("Visible"=w1003) -> ()  [unwired: 2 in, 2 out]
                n492 = property on="Hider" class="Bool (strict)"("Visible"=w1003) -> ()  [unwired: 2 in, 2 out]
              }
            }
          }
          event "ResultsAmount": Value Change {
            n493 = event-data() -> ()  [unwired: 1 in, 1 out]
            n494 = property on="ResultsSpan" class="Enum (strict)"() -> ("Value"=w1019:T16)  [unwired: 2 in, 2 out]
            n495 = Equal?(x=w1019, y=T16."Custom") -> (x = y?=w1010:bool)
            n496 = property on="ButtonRefreshResultTree" class="Bool (strict)"("Val(Sgnl)"=TRUE ("Value (Signaling)")) -> ()  [unwired: 2 in, 2 out]
            n497 = Select(t=T12."Disabled and Grayed Out" ("Disabled"), s=w1010, f=T12."Enabled" ("Disabled")) -> (s? t:f=w1015:T12)
            n498 = Select(t=T12."Enabled" ("Disabled"), s=w1010, f=T12."Disabled and Grayed Out" ("Disabled")) -> (s? t:f=w1012:T12)
            n499 = property on="ResultsAmount" class="DigNum (strict)"("DisabledEnum"=w1015) -> ()  [unwired: 2 in, 2 out]
            n500 = property on="Results.TimeFrom" class="AbsTime (strict)"("DisabledEnum"=w1012) -> (error out=w1011:errorcluster)  [unwired: 2 in, 1 out]
            n501 = case shown="True" w1010 {
              frame False {
              }
              frame True {
                n502 = invoke on="Results.TimeTo" class="AbsTime (strict)" method="Reinit To Default"() -> (error out=w1024:errorcluster)  [unwired: 3 in, 2 out]
                n503 = invoke on="Results.TimeFrom" class="AbsTime (strict)" method="Reinit To Default"(error in=w1024) -> ()  [unwired: 2 in, 3 out]
              }
            }
            n504 = property on="Results.TimeTo" class="AbsTime (strict)"(error in=w1011, "DisabledEnum"=w1012) -> ()  [unwired: 1 in, 2 out]
          }
          event "Results.TimeFrom", "Results.TimeTo": Value Change {
            w1025 = T12."Enabled" ("Disabled")
            n505 = event-data() -> ()  [unwired: 1 in, 1 out]
            n506 = property on="ButtonRefreshResultTree" class="Bool (strict)"("Val(Sgnl)"=TRUE ("Value (Signaling)")) -> ()  [unwired: 2 in, 2 out]
            n507 = property on="ResultsAmount" class="DigNum (strict)"("DisabledEnum"=T12."Disabled and Grayed Out" ("Disabled")) -> ()  [unwired: 2 in, 2 out]
            n508 = property on="ResultsSpan" class="Enum (strict)"("Value"=ProdaNG.Configurator.ResultsTimeSpan."Custom" ("ResultsSpan")) -> ()  [unwired: 2 in, 2 out]
            n509 = property on="Results.TimeFrom" class="AbsTime (strict)"("DisabledEnum"=w1025) -> (error out=w1026:errorcluster)  [unwired: 2 in, 1 out]
            n510 = property on="Results.TimeTo" class="AbsTime (strict)"(error in=w1026, "DisabledEnum"=w1025) -> ()  [unwired: 1 in, 2 out]
          }
          event "ProductListSelectAll": Value Change {
            n511 = event-data() -> ()  [unwired: 1 in, 1 out]
            n512 = case shown="\"True\"" "ProductListSelectAll" {
              tunnel: [i32[] [] ("Value (Signaling)") w1041] -> w1036
              tunnel: [enum8{"False", "True", "Mixed"}."False" ("ProductListSelectAll") enum8{"False", "True", "Mixed"}."True" ("ProductListSelectAll")] -> w1035
              frame "False", "Mixed" {
              }
              frame "True" {
                n513 = property on="ProductList" class="LstBox (strict)"() -> ("Item Names"=w1042:string[])  [unwired: 2 in, 2 out]
                n514 = for {
                  tunnel: w1042 -> [_] mode=indexing
                  tunnel: [w1044] -> w1041 mode=indexing
                  i -> [w1044]
                }
              }
            }
            n515 = property on="ProductListSelectAll" class="MixedCheckbox (strict)"("Value"=w1035) -> ()  [unwired: 2 in, 2 out]
            n516 = property on="ProductList" class="LstBox (strict)"("Val(Sgnl)"=w1036) -> ()  [unwired: 2 in, 2 out]
          }
          event "ProductList": Value Change {
            n517 = event-data() -> ()  [unwired: 1 in, 1 out]
            n518 = stacked-sequence {
              tunnel: [_ _ _ _ w1083 _] -> w1046
              tunnel: w1047 -> [_ _ _ _ w1082 _]
              tunnel: w1048 -> [_ _ _ _ w1088 _]
              tunnel: [_ _ _ _ w1084 _] -> w1045
              tunnel: [_ _ _ w1064 _ _] -> _
              frame #0 {
                w1050 = TRUE ("Value (Signaling)")
                n519 = property on="ButtonRefreshResultTree" class="Bool (strict)"("Value"=w1050) -> ()  [unwired: 2 in, 2 out]
                n520 = property on="Progress" class="Bool (strict)"("Visible"=w1050) -> ()  [unwired: 2 in, 2 out]
                n521 = property on="Hider" class="Bool (strict)"("Visible"=w1050) -> ()  [unwired: 2 in, 2 out]
              }
              frame #1 {
                n522 = local read "FPref"() -> (w1051:refnum<vi>)
                n523 = property class="Pnl"(reference=w1051, "DeferPanUpdts"=TRUE ("Defer Panel Updates")) -> ()  [unwired: 1 in, 2 out]
              }
              frame #2 {
                n524 = property on="ProductList" class="LstBox (strict)"() -> ("Item Names"=w1062:string[])  [unwired: 2 in, 2 out]
                n525 = Array Size(array=w1062) -> (size(s)=w1061:i32)
                n526 = Array Size(array="ProductList") -> (size(s)=w1060:i32)
                n527 = Equal?(x=w1060, y=w1061) -> (x = y?=w1058:bool)
                n528 = Less Or Equal To 0?(x=w1060) -> (x <= 0?=w1054:bool)
                n529 = Select(t=enum8{"False", "True", "Mixed"}."True" ("Mixed Checkbox"), s=w1058, f=enum8{"False", "True", "Mixed"}."Mixed" ("Mixed Checkbox")) -> (s? t:f=w1055:enum8{"False", "True", "Mixed"})
                n530 = Select(t=enum8{"False", "True", "Mixed"}."False" ("Mixed Checkbox"), s=w1054, f=w1055) -> (s? t:f=w1053:enum8{"False", "True", "Mixed"})
                n531 = property on="ProductListSelectAll" class="MixedCheckbox (strict)"("Value"=w1053) -> ()  [unwired: 2 in, 2 out]
              }
              frame #3 {
                w1066 = -2 ("Active Item:Row Number")
                n532 = invoke on="ResultsTree" class="Tree (strict)" method="Edit Tree Items.Delete"("tag"="", "Delete Children"=TRUE ("Delete Children?")) -> (error out=w1068:errorcluster)  [unwired: 3 in, 4 out]
                n533 = property on="ResultsTree" class="Tree (strict)"(error in=w1068, "Active Item Row Number"=w1066, "ActiveColNum"=w1066, "CellBG"=u32 16448250) -> (error out=w1067:errorcluster)  [unwired: 1 in, 1 out]
                n534 = for {
                  N: 50 -> [_]
                  tunnel: string[] ["Name", "Order", "Low Limit", "High Limit"] -> [w1076]
                  shift-right: [w1074] -> w1064
                  shift-left: w1067 -> [w1079]
                  i -> [w1073]
                  n535 = Index Array(array=w1076, index=w1073) -> (element=w1075:string)
                  n536 = property on="ResultsTree" class="Tree (strict)"(error in=w1079, "Active Item Row Number"=-1 ("Active Item:Row Number"), "ActiveColNum"=w1073, "CellBG"=u32 13816530, "Cell String"=w1075) -> (error out=w1074:errorcluster)  [unwired: 1 in, 1 out]
                }
              }
              frame #4 {
                n537 = property on="ProductList" class="LstBox (strict)" props=["Item Names", "Value"](error in=w1088) -> (error out=w1085:errorcluster, "Value"=w1089:i32[])  [unwired: 1 in, 2 out]
                n538 = local read "Products"() -> (w1081:T1[])
                n539 = for {
                  tunnel: w1081 -> [w1091]
                  tunnel: w1089 -> [w1092] mode=indexing
                  tunnel: [w1090] -> w1080 mode=indexing
                  n540 = Index Array(array=w1091, index=w1092) -> (element=w1090:T1)
                }
                n541 = local read "Identification"() -> (w1086:T7)
                n542 = control-ref of="ResultsTree"() -> (w1087:refnum<vi>)
                n543 = call "ProdaNG.Tree.Results.Update.vi"("Identification"=w1086, "Products"=w1080, "TreeControl in"=w1087, "error in (no error)"=w1085, "dbHandle in"=w1082) -> ("error out"=w1084:errorcluster, "dbHandle out"=w1083:i32)  [unwired: 4 in, 1 out]
              }
              frame #5 {
                w1093 = FALSE ("Value (Signaling)")
                n544 = property on="ButtonRefreshResultTree" class="Bool (strict)"("Value"=w1093) -> ()  [unwired: 2 in, 2 out]
                n545 = local read "FPref"() -> (w1094:refnum<vi>)
                n546 = property class="Pnl"(reference=w1094, "DeferPanUpdts"=FALSE ("Defer Panel Updates")) -> ()  [unwired: 1 in, 2 out]
                n547 = property on="Progress" class="Bool (strict)"("Visible"=w1093) -> ()  [unwired: 2 in, 2 out]
                n548 = property on="Hider" class="Bool (strict)"("Visible"=w1093) -> ()  [unwired: 2 in, 2 out]
              }
            }
          }
        }
        n549 = call <vilib>:"General Error Handler Core CORE.vi"("type of dialog (OK msg:1)"=DialogTypeEnum."continue or stop message", "error in (no error)"=w73) -> ("stop event propagated"=w69:bool, "error out"=w72:errorcluster)  [unwired: 12 in, 4 out]
        n550 = Compound Arithmetic op=OR(w69, w71) -> (w70:bool)
        n551 = call <vilib>:"Clear Errors.vi"("error in (no error)"=w72) -> ("error out"=w74:errorcluster)  [unwired: 5 in, 1 out]
      }
      n552 = call "ProdaNG.LogOut.vi"("error in"=w65, "dbHandleIn"=w66) -> ("error out"=w63:errorcluster)  [unwired: 9 in]
      n553 = call "ProdaNG.Exit.vi"("error in (no error)"=w63) -> ("error out"=w62:errorcluster)  [unwired: 10 in]
    }
    frame #3 {
      w1096 = TRUE ("Value (Signaling)")
      w1100 = -2 ("Active Item:Row Number")
      w1114 = T12."Enabled" ("Disabled")
      w1113 = FALSE ("ButtonPartList")
      w1109 = ""
      w1117 = TRUE ("Delete Children?")
      w1118 = ""
      w1107 = FALSE ("Visible")
      n554 = control-ref of="TestTree"() -> (w1121:refnum<vi>)
      n555 = invoke on="TestTree" class="Tree (strict)" method="Edit Tree Items.Delete"("tag"=w1118, "Delete Children"=w1117) -> (error out=w1120:errorcluster)  [unwired: 3 in, 4 out]
      n556 = property on="ProductList" class="LstBox (strict)"("Item Names"=string[] [], "Value"=i32[] [] ("ProductList"), "Top Row"=0) -> ()  [unwired: 2 in, 2 out]
      n557 = call "ProdaNG.Tree.Clear.vi"("TestStepsTree"=w1121) -> ()  [unwired: 10 in, 1 out]
      n558 = property on="FileInUse" class="Str"("Caption.Text"="", "Text.BGColor"=u32 13816530) -> ()  [unwired: 2 in, 2 out]
      n559 = invoke on="ProcTree" class="Tree (strict)" method="Edit Tree Items.Delete"(error in=w1120, "tag"=w1118, "Delete Children"=w1117) -> (error out=w1119:errorcluster)  [unwired: 2 in, 4 out]
      n560 = local write "Identification"(T13 {"processId"=0, "systemId"=0, "processStepId"=0, "wabcoPartId"=0} ("Identification")) -> ()
      n561 = local write "MainTab"(enum32{"Parts", "Test", "Results"}."Parts" ("MainTab")) -> ()
      n562 = property on="MainTab" class="TabCtl (strict)"("Page Labels Display Visible?"=TRUE) -> ()  [unwired: 2 in, 2 out]
      n563 = local write "DBStatus"(w1109) -> ()
      n564 = property on="ButtonRefreshResultTree" class="Bool (strict)"("Value"=w1096) -> ()  [unwired: 2 in, 2 out]
      n565 = invoke on="ResultsTree" class="Tree (strict)" method="Edit Tree Items.Delete"(error in=w1119, "tag"=w1118, "Delete Children"=w1117) -> (error out=w1098:errorcluster)  [unwired: 2 in, 4 out]
      n566 = property on="ButtonParts" class="Bool (strict)"("Value"=w1113) -> (error out=w1112:errorcluster)  [unwired: 2 in, 1 out]
      n567 = local write "Status"(w1109) -> ()
      n568 = local read "FPref"() -> (w1123:refnum<vi>)
      n569 = property on="Progress" class="Bool (strict)"("Visible"=w1107) -> ()  [unwired: 2 in, 2 out]
      n570 = property on="ButtonTest" class="Bool (strict)"(error in=w1112, "Value"=w1113, "DisabledEnum"=w1114) -> (error out=w1111:errorcluster)  [unwired: 1 in, 1 out]
      n571 = property on="ButtonRefreshTestTree" class="Bool (strict)"("Value"=w1096) -> ()  [unwired: 2 in, 2 out]
      n572 = property on="Hider" class="Bool (strict)"("Visible"=w1107) -> ()  [unwired: 2 in, 2 out]
      n573 = Close Reference(reference=w1123) -> ()  [unwired: 1 in, 1 out]
      n574 = property on="ButtonResults" class="Bool (strict)"(error in=w1111, "Value"=w1113, "DisabledEnum"=w1114) -> ()  [unwired: 1 in, 2 out]
      n575 = property on="HiderParts" class="Bool (strict)"("Visible"=w1107) -> ()  [unwired: 2 in, 2 out]
      n576 = property on="ResultsTree" class="Tree (strict)"(error in=w1098, "Active Item Row Number"=w1100, "ActiveColNum"=w1100, "CellBG"=u32 16448250) -> (error out=w1101:errorcluster)  [unwired: 1 in, 1 out]
      n577 = property on="ButtonRefreshTreeProc" class="Bool (strict)"("Value"=w1096) -> ()  [unwired: 2 in, 2 out]
      n578 = property on="ButtonConnect" class="Bool (strict)"("Value"=w1107) -> ()  [unwired: 2 in, 2 out]
      n579 = property on="ProductListSelectAll" class="MixedCheckbox (strict)"("Value"=enum8{"False", "True", "Mixed"}."False" ("Mixed Checkbox")) -> ()  [unwired: 2 in, 2 out]
      n580 = for {
        N: 50 -> [_]
        tunnel: string[] ["Name", "Order", "Low Limit", "High Limit"] -> [w1127]
        shift-right: [w1125] -> _
        shift-left: w1101 -> [w1130]
        i -> [w1124]
        n581 = Index Array(array=w1127, index=w1124) -> (element=w1126:string)
        n582 = property on="ResultsTree" class="Tree (strict)"(error in=w1130, "Active Item Row Number"=-1 ("Active Item:Row Number"), "ActiveColNum"=w1124, "CellBG"=u32 13816530, "Cell String"=w1126) -> (error out=w1125:errorcluster)  [unwired: 1 in, 1 out]
      }
      n583 = property on="Process Found" class="Bool (strict)"("Value"=w1107) -> ()  [unwired: 2 in, 2 out]
    }
    frame #4 {
      n584 = property class="App"() -> ("App.Kind"=w1133:T11)  [unwired: 2 in, 2 out]
      n585 = Equal?(x=w1133, y=T11."Run Time System") -> (x = y?=w1131:bool)
      n586 = Quit LabVIEW(quit? (T)=w1131) -> ()
    }
  }
